vi "Live Capture Functional Stack.8.64bit.vi"() -> ()   [LabVIEW 2014]
uses:
  subvis/Stack Track.ctl
  subvis/Stack_State.ctl
  CameraControlTypeDef.ctl
  Desktop/camtiff/ctiff.llb/__CTIFFNewFileAndStyleUINT16.vi
  Desktop/camtiff/ctiff.llb/__CTIFFAddNewPageUINT16.vi
panel:
  in  "Preview":bool
  in  "Capture Mode":bool
  out "Record Ready":bool
  in  "Stacks":dbl=1.0
  out "Stack Frames":i32=100
  in  "Stack Frames":i32=100
  in  "Temp":path=path "C:/temp.tmp"
  in  "Frames":i32=100
  in  "HardDisk Record":bool
  in  "Internal Line Interval":dbl
  in  "Slit Width / Lines":sgl=150.0
  in  "Camera Readout Mode":u16(ring)=12 items=["Full Frame"=1, "Slit Scanning"=12]
  in  "Readout Direction":sgl(ring)=1.0 items=["Forward"=1, "Backward"=2]
  in  "Trigger Mode":sgl(ring)=1.0 items=["Normal"=1, "Start "=6]
  in  "Trigger Source":sgl(ring)=2.0 items=["Internal"=1, "External"=2]
  out "State":T1=enum."Start Sequence"
  out "Image":u16[][](graph)
  out "Saving":bool
  in  "AutoIncrement":bool=TRUE
  in  "Path":path=path "C:/Users/spim/Desktop/Craig Cap/temp/a.tiff"
  in  "Frames":i32=100
  out "Frame Index":i32
  out "error out":errorcluster
  in  "stop":bool
  in  "Ram Record":bool
  out "Total Frames":i32
  out "Elapsed Time":u32
  out "Software FPS":dbl
  out "Camera FPS":dbl
  in  "H Offset":i32 min=0 max=0 step=4
  in  "H Width":i32 min=0 max=2048 step=4
  out "SMD":dbl
  out "SHO":i32
  in  "V Offset":i32 min=0 max=0 step=4
  in  "V Width":i32 min=0 max=2048 step=4
  in  "Binning":u16(ring) items=["1x1"=1, "2x2"=2, "4x4"=4]
  out "SHW":i32
  out "SVO":i32
  out "SVW":i32
  in  "Scan Mode":dbl min=0.0 max=2.0 step=1.0
  in  "Exposure":dbl min=0.0 max=10.000004210526315 step=1e-08
  out "EXP":dbl
  out "Camera Model":string
  out "Camera Version":string
  out "Camera Serial":string
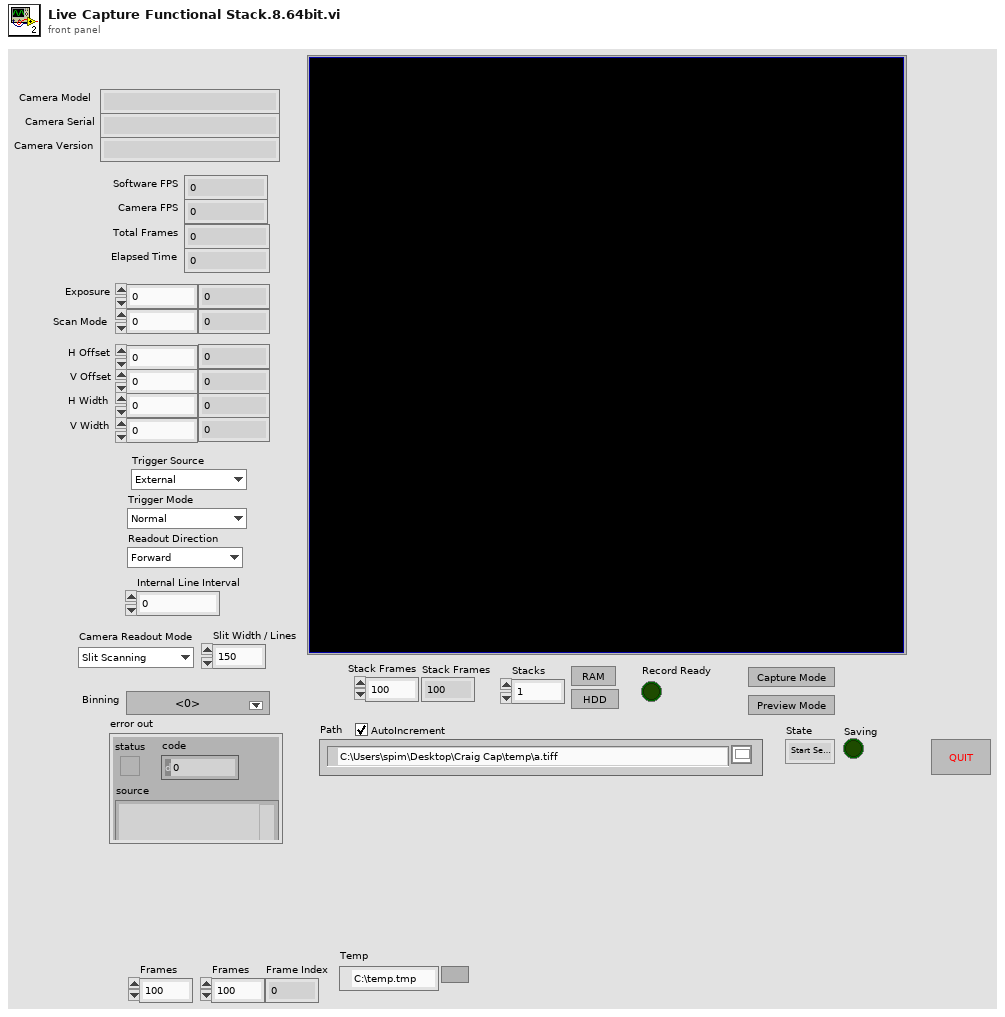
[diagram p1: front panel]
types:
  T1 = typedef "Stack Track.ctl" = enum16{"Idle", "Start Sequence", "Read Disk", "STOP", "Collecting", "End"}
  T2 = typedef "CameraControlTypeDef.ctl" = enum16{"IntervalLineInt", "Ram Record", "HardDisk Record", "Disengage Update", "Update", "Idle", "ROI", "Binning", "Scan Mode", "Trigger Mode", "Readout Mode", "Readout Direction", "Preview"}
  T3 = typedef "Stack_State.ctl" = cluster{"State":T1, "Stack Number":i32, "Image":u16[][]}
  T4 = enum8{"Enabled", "Disabled", "Disabled and Grayed Out"}
  T5 = cluster{"Model":string, "Camera ID":string, "Firmware":string}
  T6 = cluster{"Value":i32, "Minimum":i32, "Maximum":i32, "Increment":i32}
  T7 = cluster{"height":u32, "width":u32, "datatype":u32}
  T8 = cluster{"H Offset":i32, "V Offset":i32, "H Width":i32, "V Width":i32}
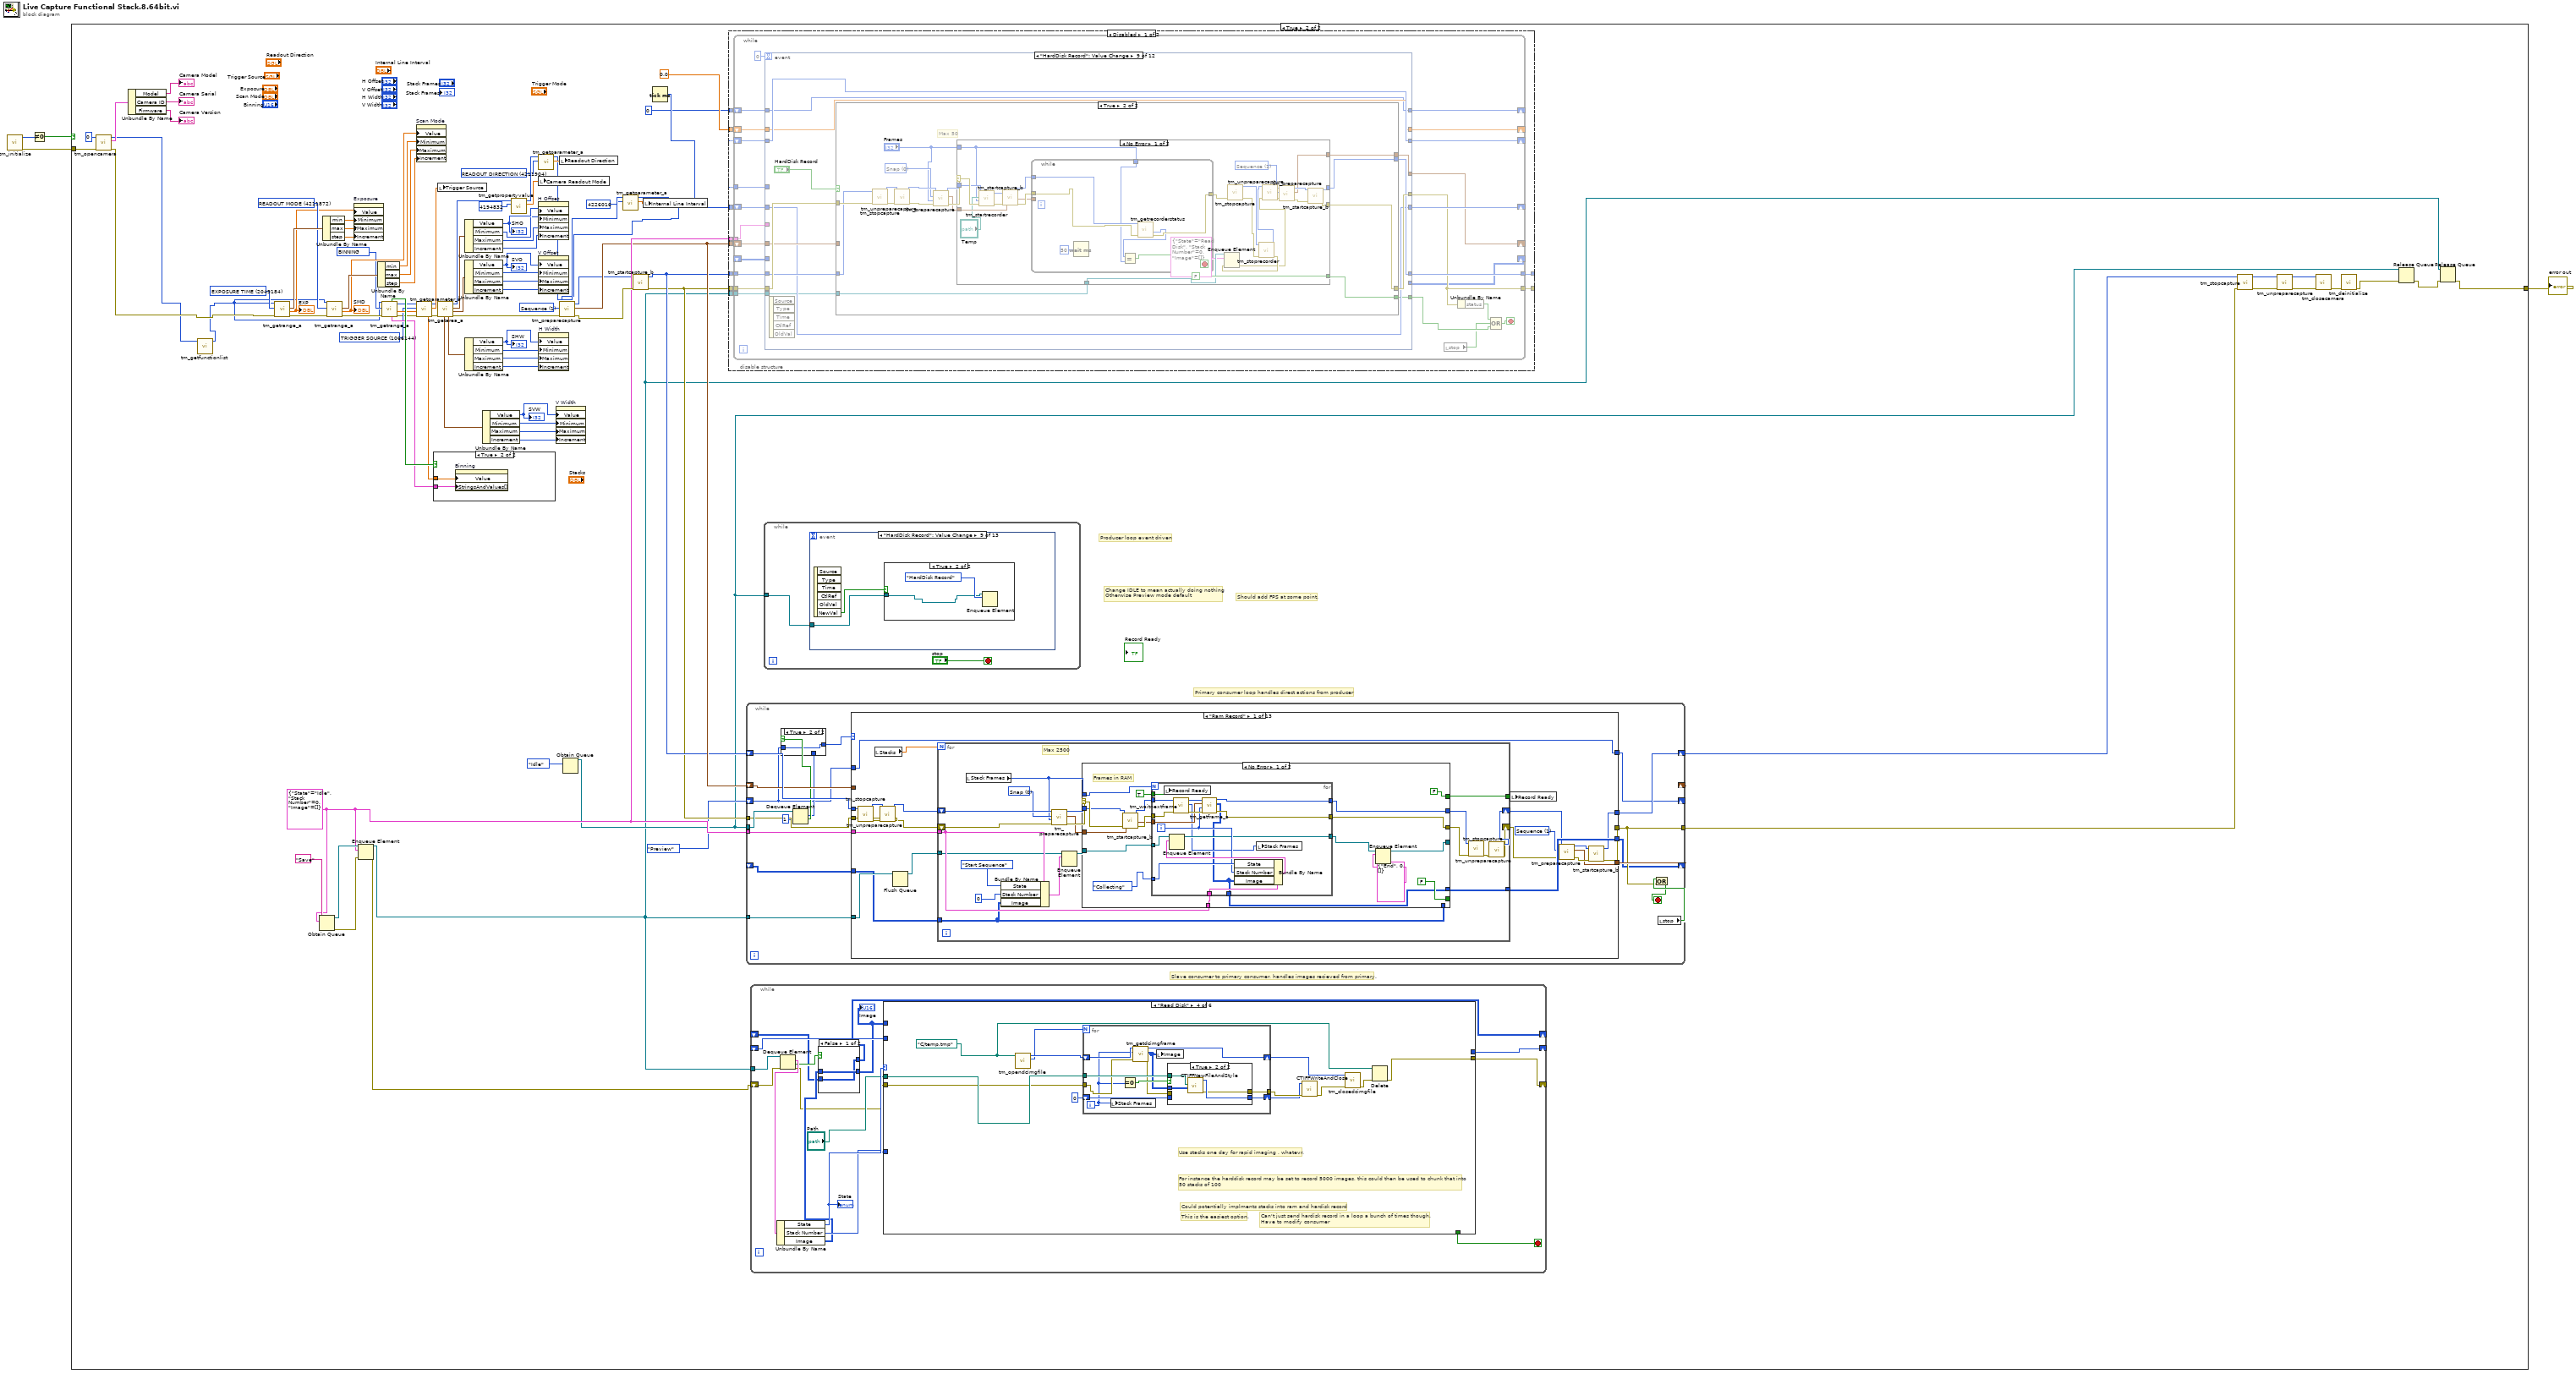
[diagram p0: block diagram]
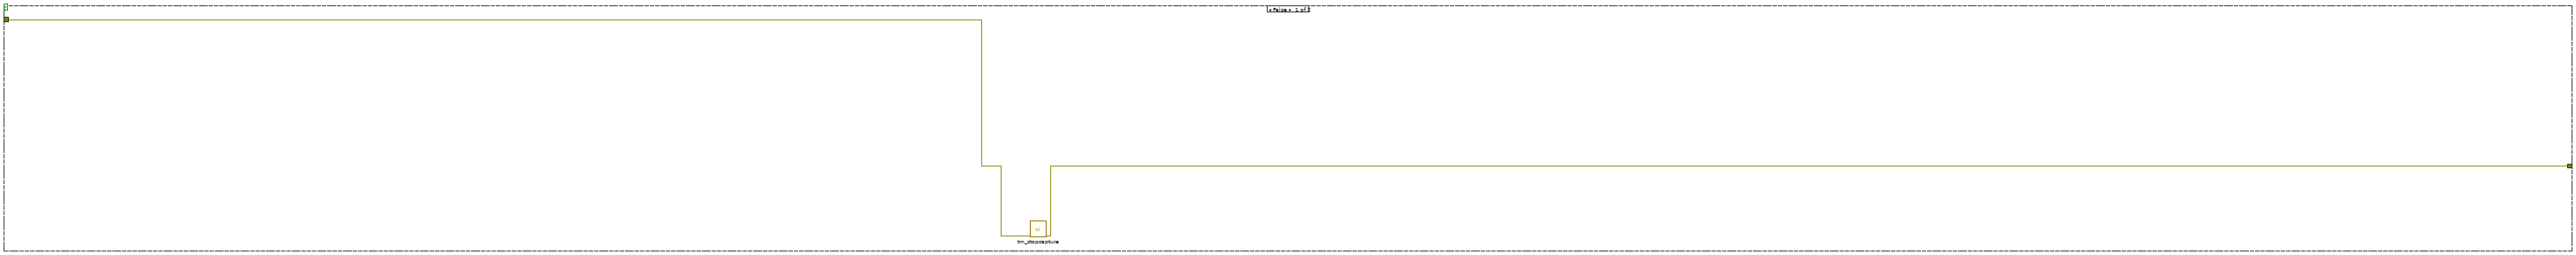
[diagram p2: hidden frame]
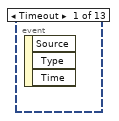
[diagram p3: hidden frame]
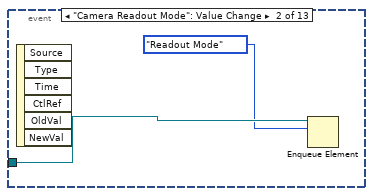
[diagram p4: hidden frame]
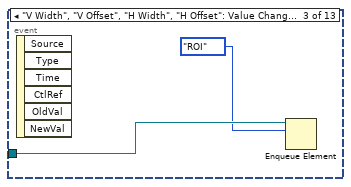
[diagram p5: hidden frame]
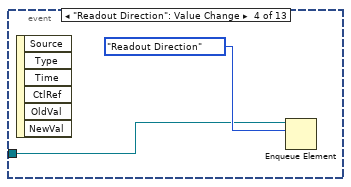
[diagram p6: hidden frame]
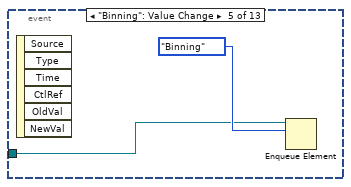
[diagram p7: hidden frame]
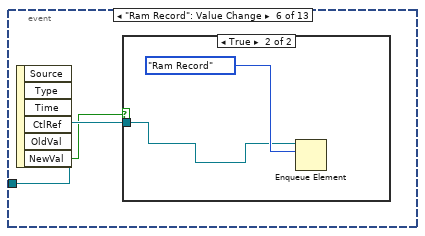
[diagram p8: hidden frame]
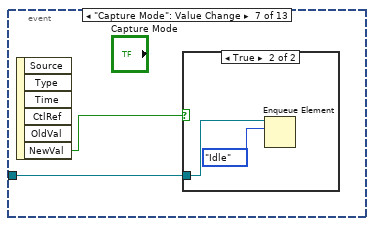
[diagram p10: hidden frame]
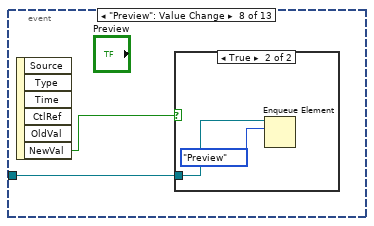
[diagram p12: hidden frame]
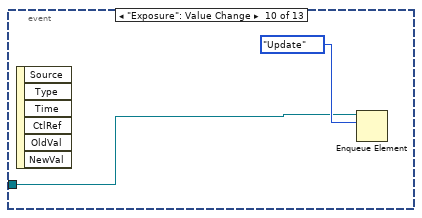
[diagram p15: hidden frame]
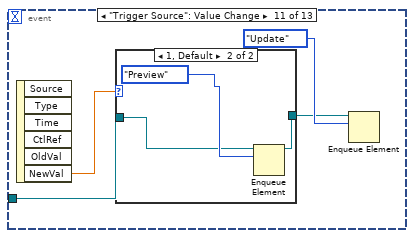
[diagram p16: hidden frame]
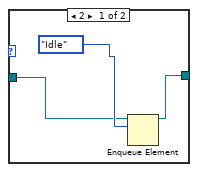
[diagram p17: hidden frame]
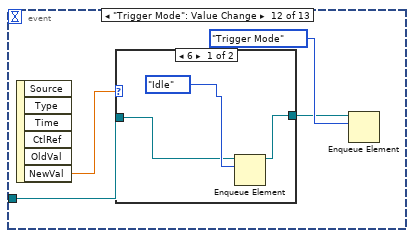
[diagram p18: hidden frame]
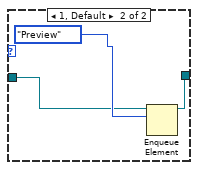
[diagram p19: hidden frame]
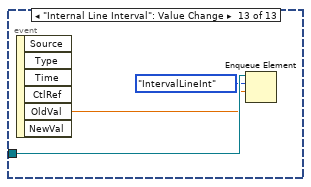
[diagram p20: hidden frame]
diagram:
  n1 = call <userlib>:"tm_initialize.vi"() -> ("error out"=w2:errorcluster, "Number Of Cameras"=w1:u32)  [unwired: 8 in, 2 out]
  n2 = Not Equal To 0?(x=w1) -> (x != 0?=w4:bool)
  n3 = case shown="True" w4 {
    tunnel: [w5 w15] -> w3
    tunnel: w2 -> [w6 w98]
    frame False {
      n4 = call <userlib>:"tm_stopcapture.vi"("error in (no error)"=w6) -> ("error out"=w5:errorcluster)  [unwired: 9 in, 1 out]
    }
    frame True {
      w33 = u32 4211904 items=["SENSOR MODE"=4212128, "CCD MODE"=4212384, "READOUT MODE"=4211872, "ACTIVE VIEW INDEX"=4343136, "BITS PER CHANNEL"=4342976, "IMAGE PIXEL TYPE"=4343296, "BINNING"=4215968, "EXPOSURE TIME"=2049184, "CONTRAST GAIN"=3163312, "CONTRAST OFFSET"=3163328, "LIGHT MODE"=2114720, "SENSITIVITY"=2114992, "PHOTON IMAGING MODE"=2115200, "HIGH DYNAMIC RANGE MODE"=3163360, "WHITE BALANCE"=3163568, "TEMPERATURE"=2115232, "TEMPERATURE TARGET"=2115264, "SENSOR COOLER FAN"=2115296, "LINEBUNDLE HEIGHT"=4212192, "MECHANICAL SHUTTER"=2115488, "BACK FOCUS POSITION"=8422304, "TRIGGER CONNECTOR"=1066432, "TRIGGER SOURCE"=1066144, "OUTPUT TRIGGER SOURCE"=1852576, "TRIGGER GLOBAL EXPOSURE"=2049680, "FIRST TRIGGER BEHAVIOR"=2049696, "CHANNEL SYNC"=1852352, "READOUT DIRECTION"=4211904, "PRE HSYNC COUNT"=1852704] ("Parameter")
      w42 = u32 1066144 items=["SENSOR MODE"=4212128, "CCD MODE"=4212384, "READOUT MODE"=4211872, "ACTIVE VIEW INDEX"=4343136, "BITS PER CHANNEL"=4342976, "IMAGE PIXEL TYPE"=4343296, "BINNING"=4215968, "EXPOSURE TIME"=2049184, "CONTRAST GAIN"=3163312, "CONTRAST OFFSET"=3163328, "LIGHT MODE"=2114720, "SENSITIVITY"=2114992, "PHOTON IMAGING MODE"=2115200, "HIGH DYNAMIC RANGE MODE"=3163360, "WHITE BALANCE"=3163568, "TEMPERATURE"=2115232, "TEMPERATURE TARGET"=2115264, "SENSOR COOLER FAN"=2115296, "LINEBUNDLE HEIGHT"=4212192, "MECHANICAL SHUTTER"=2115488, "BACK FOCUS POSITION"=8422304, "TRIGGER CONNECTOR"=1066432, "TRIGGER SOURCE"=1066144, "OUTPUT TRIGGER SOURCE"=1852576, "TRIGGER GLOBAL EXPOSURE"=2049680, "FIRST TRIGGER BEHAVIOR"=2049696, "CHANNEL SYNC"=1852352, "READOUT DIRECTION"=4211904, "PRE HSYNC COUNT"=1852704] ("Parameter")
      w28 = T3 {"State"=enum."Idle", "Stack Number"=0, "Image"=[]} ("input cluster")
      w47 = u32 2049184 items=["BINNING"=4215968, "BITS PER CHANNEL"=4342976, "ACTIVE VIEW INDEX"=4343136, "CCD MODE"=4212384, "SENSOR MODE"=4212128, "READOUT MODE"=4211872, "EXPOSURE TIME"=2049184, "CONTRAST GAIN"=3163312, "CONTRAST OFFSET"=3163328, "LIGHT MODE"=2114720, "SENSITIVITY"=2114992, "WHITE BALANCE"=3163568, "PHOTON IMAGING MODE"=2115200, "HIGH DYNAMIC RANGE MODE"=3163360, "TRIGGER SOURCE"=1066144, "TRIGGER ACTIVE"=1066160, "TRIGGER MODE"=1066400, "TRIGGER POLARITY"=1066416, "TRIGGER GLOBAL EXPOSURE"=2049680, "FIRST TRIGGER BEHAVIOR"=2049696, "TRIGGER TIMES"=1066448, "OUTPUT TRIGGER POLARITY"=1852592, "OUTPUT TRIGGER DELAY"=1852624, "OUTPUT TRIGGER PERIOD"=1852640, "TEMPERATURE"=2115232, "TEMPERATURE TARGET"=2115264, "SENSOR COOLER FAN"=2115296, "MECHANICAL SHUTTER"=2115488, "BACK FOCUS POSITION"=8422304, "FRAMEBUNDLE MODE"=4346784, "FRAMEBUNDLE NUMBER"=4346800, "LINEBUNDLE HEIGHT"=4212192, "TRIGGER CONNECTOR"=1066432, "IMAGE PIXEL TYPE"=4343296, "OUTPUT TRIGGER KIND"=1852656, "READOUT DIRECTION"=4211904, "CHANNEL SYNC"=1852352] ("Parameter")
      w48 = u32 4211872 items=["BINNING"=4215968, "BITS PER CHANNEL"=4342976, "ACTIVE VIEW INDEX"=4343136, "CCD MODE"=4212384, "SENSOR MODE"=4212128, "READOUT MODE"=4211872, "EXPOSURE TIME"=2049184, "CONTRAST GAIN"=3163312, "CONTRAST OFFSET"=3163328, "LIGHT MODE"=2114720, "SENSITIVITY"=2114992, "WHITE BALANCE"=3163568, "PHOTON IMAGING MODE"=2115200, "HIGH DYNAMIC RANGE MODE"=3163360, "TRIGGER SOURCE"=1066144, "TRIGGER ACTIVE"=1066160, "TRIGGER MODE"=1066400, "TRIGGER POLARITY"=1066416, "TRIGGER GLOBAL EXPOSURE"=2049680, "FIRST TRIGGER BEHAVIOR"=2049696, "TRIGGER TIMES"=1066448, "OUTPUT TRIGGER POLARITY"=1852592, "OUTPUT TRIGGER DELAY"=1852624, "OUTPUT TRIGGER PERIOD"=1852640, "TEMPERATURE"=2115232, "TEMPERATURE TARGET"=2115264, "SENSOR COOLER FAN"=2115296, "MECHANICAL SHUTTER"=2115488, "BACK FOCUS POSITION"=8422304, "FRAMEBUNDLE MODE"=4346784, "FRAMEBUNDLE NUMBER"=4346800, "LINEBUNDLE HEIGHT"=4212192, "TRIGGER CONNECTOR"=1066432, "IMAGE PIXEL TYPE"=4343296, "OUTPUT TRIGGER KIND"=1852656, "READOUT DIRECTION"=4211904, "CHANNEL SYNC"=1852352] ("Parameter")
      w49 = u32 4215968 items=["BINNING"=4215968, "BITS PER CHANNEL"=4342976, "ACTIVE VIEW INDEX"=4343136, "CCD MODE"=4212384, "SENSOR MODE"=4212128, "READOUT MODE"=4211872, "EXPOSURE TIME"=2049184, "CONTRAST GAIN"=3163312, "CONTRAST OFFSET"=3163328, "LIGHT MODE"=2114720, "SENSITIVITY"=2114992, "WHITE BALANCE"=3163568, "PHOTON IMAGING MODE"=2115200, "HIGH DYNAMIC RANGE MODE"=3163360, "TRIGGER SOURCE"=1066144, "TRIGGER ACTIVE"=1066160, "TRIGGER MODE"=1066400, "TRIGGER POLARITY"=1066416, "TRIGGER GLOBAL EXPOSURE"=2049680, "FIRST TRIGGER BEHAVIOR"=2049696, "TRIGGER TIMES"=1066448, "OUTPUT TRIGGER POLARITY"=1852592, "OUTPUT TRIGGER DELAY"=1852624, "OUTPUT TRIGGER PERIOD"=1852640, "TEMPERATURE"=2115232, "TEMPERATURE TARGET"=2115264, "SENSOR COOLER FAN"=2115296, "MECHANICAL SHUTTER"=2115488, "BACK FOCUS POSITION"=8422304, "FRAMEBUNDLE MODE"=4346784, "FRAMEBUNDLE NUMBER"=4346800, "LINEBUNDLE HEIGHT"=4212192, "TRIGGER CONNECTOR"=1066432, "IMAGE PIXEL TYPE"=4343296, "OUTPUT TRIGGER KIND"=1852656, "READOUT DIRECTION"=4211904, "CHANNEL SYNC"=1852352] ("Parameter")
      w94 = 1 items=["Snap", "Sequence"] ("Capture mode")
      # "Change IDLE to mean actually doing nothing\nOtherwise Preview mode default"
      # "Slave consumer to primary consumer, handles images recieved from primary."
      # "Primary consumer loop handles direct actions from producer"
      # "Producer loop event driven"
      # "Should add FPS at some point."
      n5 = call <userlib>:"tm_opencamera.vi"("error in (no error)"=w98, "Camera Index"=u32 0) -> ("error out"=w29:errorcluster, "Camera Details"=w61:T5, "Handle out"=w13:u32)  [unwired: 7 in]
      n6 = Unbundle By Name(w61) -> ("Model"=→"Camera Model":string, "Camera ID"=→"Camera Serial":string, "Firmware"=→"Camera Version":string)
      n7 = call <userlib>:"tm_getfunctionlist.vi"("Handle in"=w13) -> ("Handle out"=w12:u32)  [unwired: 8 in, 2 out]
      n8 = call <userlib>:"tm_getrange_a.vi"("error in (no error)"=w29, "Parameter"=w47, "Handle in"=w12) -> ("error out"=w56:errorcluster, "default"=w45:dbl, "Range"=w57:cluster{"min":dbl, "max":dbl, "step":dbl})  [unwired: 2 in, 4 out]
      "EXP" <- w45
      n9 = Obtain Queue(name (unnamed)="Save", element data type=w28) -> (queue out=w31:refnum<queue>, error out=w10:errorcluster)  [unwired: 3 in, 1 out]
      n10 = Unbundle By Name(w57) -> ("min"=w92:dbl, "max"=w91:dbl, "step"=w90:dbl)
      n11 = call <userlib>:"tm_getrange_a.vi"("error in (no error)"=w56, "Parameter"=w48, "Handle in"=w12) -> ("error out"=w53:errorcluster, "default"=w54:dbl, "Range"=w55:cluster{"min":dbl, "max":dbl, "step":dbl})  [unwired: 2 in, 4 out]
      "SMD" <- w54
      n12 = property on="Exposure" class="DigNum (strict)"("Value"=w45, "Minimum"=w92, "Maximum"=w91, "Increment"=w90) -> ()  [unwired: 2 in, 2 out]
      n13 = Enqueue Element(queue=w31, element=w28, error in (no error)=w10) -> (queue out=w14:refnum<queue>, error out=w9:errorcluster)  [unwired: 1 in, 1 out]
      n14 = Unbundle By Name(w55) -> ("min"=w89:dbl, "max"=w88:dbl, "step"=w87:dbl)
      n15 = call <userlib>:"tm_getrange_a.vi"("error in (no error)"=w53, "Parameter"=w49, "Handle in"=w12) -> ("error out"=w39:errorcluster, "default"=w51:dbl, "Handle out"=w41:u32, "Value Names"=w50:cluster{"Name":string, "Value":dbl}[], "Writable"=w52:bool)  [unwired: 2 in, 2 out]
      n16 = property on="Scan Mode" class="DigNum (strict)"("Value"=w54, "Minimum"=w89, "Maximum"=w88, "Increment"=w87) -> ()  [unwired: 2 in, 2 out]
      n17 = call <userlib>:"tm_getparameter_a.vi"("error in (no error)"=w39, "Parameter"=w42, "Handle in"=w41) -> ("error out"=w38:errorcluster, "Value out"=w43:dbl, "Handle out"=w40:u32)  [unwired: 6 in]
      n18 = case shown="True" w52 {
        tunnel: w50 -> [_ w1167]
        tunnel: w51 -> [_ w1166]
        frame False {
        }
        frame True {
          n19 = property on="Binning" class="Ring (strict)"("Value"=w1166, "StringsAndValues[]"=w1167) -> ()  [unwired: 2 in, 2 out]
        }
      }
      n20 = local write "Trigger Source"(w43) -> ()
      n21 = call <userlib>:"tm_getarea_a.vi"("error in (no error)"=w38, "Handle in"=w40) -> ("error out"=w44:errorcluster, "V Offset"=w86:T6, "H Offset"=w67:T6, "Handle out"=w35:u32, "H Width"=w85:T6, "V Width"=w84:T6)  [unwired: 4 in]
      n22 = Unbundle By Name(w67) -> ("Value"=w66:i32, "Minimum"=w65:i32, "Maximum"=w64:i32, "Increment"=w63:i32)
      "SHO" <- w66
      n23 = Unbundle By Name(w86) -> ("Value"=w74:i32, "Minimum"=w83:i32, "Maximum"=w82:i32, "Increment"=w81:i32)
      "SVO" <- w74
      n24 = Unbundle By Name(w85) -> ("Value"=w73:i32, "Minimum"=w80:i32, "Maximum"=w79:i32, "Increment"=w78:i32)
      "SHW" <- w73
      n25 = Unbundle By Name(w84) -> ("Value"=w72:i32, "Minimum"=w77:i32, "Maximum"=w76:i32, "Increment"=w75:i32)
      "SVW" <- w72
      n26 = call <userlib>:"tm_getpropertyvalue.vi"("Property ID"=u32 4194832, "Handle in"=w35) -> ("Value in"=w36:sgl, "Handle out"=w34:u32)  [unwired: 7 in, 1 out]
      n27 = call <userlib>:"tm_getparameter_a.vi"("Parameter"=w33, "Handle in"=w34) -> ("Value out"=w32:dbl, "Handle out"=w19:u32)  [unwired: 7 in, 1 out]
      n28 = local write "Camera Readout Mode"(w36) -> ()
      n29 = property on="H Offset" class="DigNum (strict)"("Value"=w66, "Minimum"=w65, "Maximum"=w64, "Increment"=w63) -> ()  [unwired: 2 in, 2 out]
      n30 = property on="V Offset" class="DigNum (strict)"("Value"=w74, "Minimum"=w83, "Maximum"=w82, "Increment"=w81) -> ()  [unwired: 2 in, 2 out]
      n31 = property on="H Width" class="DigNum (strict)"("Value"=w73, "Minimum"=w80, "Maximum"=w79, "Increment"=w78) -> ()  [unwired: 2 in, 2 out]
      n32 = property on="V Width" class="DigNum (strict)"("Value"=w72, "Minimum"=w77, "Maximum"=w76, "Increment"=w75) -> ()  [unwired: 2 in, 2 out]
      n33 = local write "Readout Direction"(w32) -> ()
      n34 = Obtain Queue(element data type=CameraControlTypeDef."Idle" ("Enum")) -> (queue out=w17:refnum<queue>)  [unwired: 4 in, 2 out]
      n35 = call <userlib>:"tm_getparameter_a.vi"("Parameter"=4226016, "Handle in"=w19) -> ("Value out"=w7:dbl, "Handle out"=w8:u32)  [unwired: 7 in, 1 out]
      n36 = call <userlib>:"tm_preparecapture.vi"("error in (no error)"=w44, "Capture mode"=w94, "Handle in"=w8) -> ("error out"=w30:errorcluster, "Buffer Info"=w27:T7, "Handle out"=w20:u32)  [unwired: 5 in, 1 out]
      n37 = call <userlib>:"tm_startcapture_b.vi"("error in (no error)"=w30, "Handle in"=w20) -> ("error out"=w25:errorcluster, "Handle out"=w26:u32)  [unwired: 8 in]
      n38 = local write "Internal Line Interval"(w7) -> ()
      n39 = Tick Count (ms)() -> (millisecond timer value=w93:u32)
      n40 = disable-structure shown="Disabled" {
        disable-tunnel: 0.0 -> [w582 _]
        disable-tunnel: w93 -> [w581 _]
        disable-tunnel: 0 -> [w580 _]
        disable-tunnel: [w579 _] -> _
        disable-tunnel: [w578 _] -> _
        disable-tunnel: w28 -> [w577 _]
        disable-tunnel: w27 -> [w576 _]
        disable-tunnel: w26 -> [w575 _]
        disable-tunnel: w25 -> [w574 _]
        disable-tunnel: w14 -> [w573 _]
        frame Disabled {
          n41 = while {
            tunnel: w574 -> [w596]
            tunnel: [w594] -> w578
            tunnel: [w593] -> w579
            shift-right: [w603] -> _
            shift-left: w581 -> [w601]
            shift-right: [w604] -> _
            shift-left: w582 -> [w602]
            shift-right: [w595] -> _
            shift-left: w581 -> [w599]
            tunnel: w575 -> [w597]
            tunnel: w581 -> [w600]
            shift-right: [w592] -> _
            shift-left: w576 -> [w598]
            shift-right: [w590] -> _
            shift-left: w580 -> [w591]
            tunnel: w573 -> [w589]
            shift-right: [w587] -> _
            shift-left: _ -> [w586]
            tunnel: w577 -> [w585]
            stop <- w605 stop-if-true
            n42 = event shown="[8] \"HardDisk Record\": Value Change" {
              selector: _ -> [_ _ _ _ _ _ _ _ _ _ _ _]
              dyn-events: _ -> [_ _ _ _ _ _ _ _ _ _ _ _]
              timeout: 0 -> [_ _ _ _ _ _ _ _ _ _ _ _]
              tunnel: [w616 w685 w699 w712 w731 w751 w773 w801 w898 w992 w1028 w1073] -> w604
              tunnel: [w615 w686 w700 w713 w732 w752 w774 w802 w899 w993 w1029 w1074] -> w603
              tunnel: w602 -> [w627 w685 w699 w712 w731 w751 w773 w801 w898 w992 w1028 w1073]
              tunnel: w601 -> [w618 w686 w700 w713 w732 w752 w774 w802 w899 w993 w1029 w1074]
              tunnel: w600 -> [w623 _ _ _ _ _ _ _ _ _ _ _]
              tunnel: w599 -> [w628 w687 w701 w714 w733 w753 w775 w797 w894 w994 w1036 w1081]
              tunnel: w598 -> [w622 w684 w698 w711 _ w750 _ w798 w895 _ _ _]
              tunnel: w597 -> [w630 w680 w693 w707 w726 w744 w766 w805 w902 w989 w1005 w1043]
              tunnel: w596 -> [w629 w682 w689 w708 w725 w747 w765 w806 w903 w988 w1004 w1042]
              tunnel: [w626 w687 w701 w714 w733 w753 w775 w797 w894 w994 w1036 w1081] -> w595
              tunnel: [w625 w677 w696 w704 w717 w737 w756 w803 w900 w983 w1031 w1076] -> w594
              tunnel: [w624 w676 w695 w703 w716 w736 w754 w804 w901 w984 w1032 w1077] -> w593
              tunnel: [w621 w684 w698 w711 w720 w750 w761 w799 w896 w982 w1030 w1075] -> w592
              tunnel: w591 -> [w613 w683 w697 w710 w730 w749 w772 w800 w897 w981 w1001 w1037]
              tunnel: [w612 w683 w697 w710 w730 w749 w772 w800 w897 w981 w1001 w1037] -> w590
              tunnel: w589 -> [w607 _ _ _ _ _ _ w796 w893 _ _ _]
              tunnel: [_ _ _ _ _ _ _ w795 w892 _ _ _] -> w588
              tunnel: w585 -> [w610 _ _ _ _ _ _ w793 _ _ _ _]
              tunnel: [w609 _ _ _ _ _ _ _ _ _ _ _] -> w587
              tunnel: w586 -> [w608 _ _ _ _ _ _ w794 _ _ _ _]
              event Timeout {
                n43 = event-data() -> ()  [unwired: 1 in, 2 out]
                n44 = call <userlib>:"tm_waitnextframe.vi"("error in (no error)"=w629, "Handle in"=w630) -> ("error out"=w633:errorcluster, "Frame Count"=w614:i32, "Frame Index"=w632:i32, "Handle out"=w634:u32)  [unwired: 6 in]
                "Total Frames" <- w614
                n45 = Tick Count (ms)() -> (millisecond timer value=w620:u32)
                n46 = Increment(x=w627) -> (x+1=w617:dbl)
                n47 = Subtract(x=w620, y=w623) -> (x-y=→"Elapsed Time":u32)
                n48 = Add(x=w618, y=u32 1000) -> (x+y=w638:u32)
                n49 = Less Or Equal?(x=w638, y=w620) -> (x <= y?=w619:bool)
                n50 = Add(x=w628, y=u32 50) -> (x+y=w636:u32)
                n51 = Less Or Equal?(x=w636, y=w620) -> (x <= y?=w611:bool)
                n52 = case shown="True" w619 {
                  tunnel: w618 -> [w641 w650]
                  tunnel: [w641 w647] -> w615
                  tunnel: w617 -> [w640 w653]
                  tunnel: w620 -> [_ w647]
                  tunnel: [w640 0.0] -> w616
                  tunnel: w614 -> [_ w642]
                  tunnel: w613 -> [w639 w645]
                  tunnel: [w639 w642] -> w612
                  frame False {
                  }
                  frame True {
                    n53 = Subtract(x=w647, y=w650) -> (x-y=w649:u32)
                    n54 = Subtract(x=w642, y=w645) -> (x-y=w643:i32)
                    n55 = To Double Precision Float(number=w649) -> (double precision float=w655:dbl)
                    n56 = Divide(x=w655, y=1000.0) -> (x/y=w646:dbl)
                    n57 = To Double Precision Float(number=w643) -> (double precision float=w644:dbl)
                    n58 = Divide(x=w644, y=w646) -> (x/y=→"Camera FPS":dbl)
                    n59 = Divide(x=w653, y=w646) -> (x/y=→"Software FPS":dbl)
                  }
                }
                n60 = case shown="True" w611 {
                  tunnel: w628 -> [w660 _]
                  tunnel: w620 -> [_ w673]
                  tunnel: [w660 w673] -> w626
                  tunnel: w634 -> [w659 w672]
                  tunnel: w622 -> [w657 w667]
                  tunnel: w633 -> [w658 w671]
                  tunnel: [w659 w670] -> w625
                  tunnel: [w658 w669] -> w624
                  tunnel: w632 -> [_ w668]
                  tunnel: [w657 w667] -> w621
                  tunnel: w607 -> [_ w666]
                  tunnel: w610 -> [_ w662]
                  tunnel: [w656 w661] -> w609
                  tunnel: w608 -> [w656 _]
                  frame False {
                  }
                  frame True {
                    n61 = call <userlib>:"tm_getframe_a.vi"("error in (no error)"=w671, "Frame Index"=w668, "Buffer Info"=w667, "Handle in"=w672) -> ("error out"=w669:errorcluster, "Data 16"=w661:u16[][], "Handle out"=w670:u32)  [unwired: 3 in, 2 out]
                    n62 = Bundle By Name(cluster=w662, "State"=Stack_Track."Idle", "Stack Number"=0, "Image"=w661) -> (w663:T3)
                    n63 = Enqueue Element(queue=w666, element=w663) -> ()  [unwired: 2 in, 3 out]
                  }
                }
              }
              event "Exposure": Value Change {
                w675 = u32 2049184 items=["SENSOR MODE"=4212128, "CCD MODE"=4212384, "READOUT MODE"=4211872, "ACTIVE VIEW INDEX"=4343136, "BITS PER CHANNEL"=4342976, "IMAGE PIXEL TYPE"=4343296, "BINNING"=4215968, "EXPOSURE TIME"=2049184, "CONTRAST GAIN"=3163312, "CONTRAST OFFSET"=3163328, "LIGHT MODE"=2114720, "SENSITIVITY"=2114992, "PHOTON IMAGING MODE"=2115200, "HIGH DYNAMIC RANGE MODE"=3163360, "WHITE BALANCE"=3163568, "TEMPERATURE"=2115232, "TEMPERATURE TARGET"=2115264, "SENSOR COOLER FAN"=2115296, "LINEBUNDLE HEIGHT"=4212192, "MECHANICAL SHUTTER"=2115488, "BACK FOCUS POSITION"=8422304, "TRIGGER CONNECTOR"=1066432, "TRIGGER SOURCE"=1066144, "OUTPUT TRIGGER SOURCE"=1852576, "TRIGGER GLOBAL EXPOSURE"=2049680, "FIRST TRIGGER BEHAVIOR"=2049696, "CHANNEL SYNC"=1852352, "READOUT DIRECTION"=4211904, "PRE HSYNC COUNT"=1852704] ("Parameter")
                n64 = event-data() -> ("NewVal"=w681:dbl)  [unwired: 1 in, 2 out]
                n65 = call <userlib>:"tm_setparameter_a.vi"("error in (no error)"=w682, "Value in"=w681, "Parameter"=w675, "Handle in"=w680) -> ("error out"=w679:errorcluster, "Handle out"=w678:u32)  [unwired: 6 in]
                n66 = call <userlib>:"tm_getparameter_a.vi"("error in (no error)"=w679, "Parameter"=w675, "Handle in"=w678) -> ("error out"=w676:errorcluster, "Value out"=w674:dbl, "Handle out"=w677:u32)  [unwired: 6 in]
                n67 = local write "EXP"(w674) -> ()
              }
              event "Internal Line Interval": Value Change {
                w688 = u32 4191424 items=["SENSOR MODE"=4212128, "CCD MODE"=4212384, "READOUT MODE"=4211872, "ACTIVE VIEW INDEX"=4343136, "BITS PER CHANNEL"=4342976, "IMAGE PIXEL TYPE"=4343296, "BINNING"=4215968, "EXPOSURE TIME"=2049184, "CONTRAST GAIN"=3163312, "CONTRAST OFFSET"=3163328, "LIGHT MODE"=2114720, "SENSITIVITY"=2114992, "PHOTON IMAGING MODE"=2115200, "HIGH DYNAMIC RANGE MODE"=3163360, "WHITE BALANCE"=3163568, "TEMPERATURE"=2115232, "TEMPERATURE TARGET"=2115264, "SENSOR COOLER FAN"=2115296, "LINEBUNDLE HEIGHT"=4212192, "MECHANICAL SHUTTER"=2115488, "BACK FOCUS POSITION"=8422304, "TRIGGER CONNECTOR"=1066432, "TRIGGER SOURCE"=1066144, "OUTPUT TRIGGER SOURCE"=1852576, "TRIGGER GLOBAL EXPOSURE"=2049680, "FIRST TRIGGER BEHAVIOR"=2049696, "CHANNEL SYNC"=1852352, "READOUT DIRECTION"=4211904, "PRE HSYNC COUNT"=1852704, "INTERNAL LINE SPEED"=4191408, "INTERNAL LINE INVERVAL"=4191424] ("Parameter")
                n68 = event-data() -> ("NewVal"=w692:dbl)  [unwired: 1 in, 2 out]
                n69 = call <userlib>:"tm_setparameter_a.vi"("error in (no error)"=w689, "Value in"=w692, "Parameter"=w688, "Handle in"=w693) -> ("error out"=w690:errorcluster, "Handle out"=w691:u32)  [unwired: 6 in]
                n70 = call <userlib>:"tm_getparameter_a.vi"("error in (no error)"=w690, "Parameter"=w688, "Handle in"=w691) -> ("error out"=w695:errorcluster, "Value out"=w694:dbl, "Handle out"=w696:u32)  [unwired: 6 in]
                n71 = local write "Internal Line Interval"(w694) -> ()
              }
              event "Trigger Source": Value Change {
                w709 = u32 1066144 items=["SENSOR MODE"=4212128, "CCD MODE"=4212384, "READOUT MODE"=4211872, "ACTIVE VIEW INDEX"=4343136, "BITS PER CHANNEL"=4342976, "IMAGE PIXEL TYPE"=4343296, "BINNING"=4215968, "EXPOSURE TIME"=2049184, "CONTRAST GAIN"=3163312, "CONTRAST OFFSET"=3163328, "LIGHT MODE"=2114720, "SENSITIVITY"=2114992, "PHOTON IMAGING MODE"=2115200, "HIGH DYNAMIC RANGE MODE"=3163360, "WHITE BALANCE"=3163568, "TEMPERATURE"=2115232, "TEMPERATURE TARGET"=2115264, "SENSOR COOLER FAN"=2115296, "LINEBUNDLE HEIGHT"=4212192, "MECHANICAL SHUTTER"=2115488, "BACK FOCUS POSITION"=8422304, "TRIGGER CONNECTOR"=1066432, "TRIGGER SOURCE"=1066144, "OUTPUT TRIGGER SOURCE"=1852576, "TRIGGER GLOBAL EXPOSURE"=2049680, "FIRST TRIGGER BEHAVIOR"=2049696, "CHANNEL SYNC"=1852352, "READOUT DIRECTION"=4211904, "PRE HSYNC COUNT"=1852704] ("Parameter")
                n72 = event-data() -> ("NewVal"=w702:sgl)  [unwired: 1 in, 3 out]
                n73 = call <userlib>:"tm_setparameter_a.vi"("error in (no error)"=w708, "Value in"=w702, "Parameter"=w709, "Handle in"=w707) -> ("error out"=w706:errorcluster, "Handle out"=w705:u32)  [unwired: 6 in]
                n74 = call <userlib>:"tm_getparameter_a.vi"("error in (no error)"=w706, "Parameter"=w709, "Handle in"=w705) -> ("error out"=w703:errorcluster, "Handle out"=w704:u32)  [unwired: 6 in, 1 out]
              }
              event "Trigger Mode": Value Change {
                w721 = 1 items=["Snap", "Sequence"] ("Capture mode")
                n75 = event-data() -> ("NewVal"=w715:sgl)  [unwired: 1 in, 4 out]
                n76 = call <userlib>:"tm_stopcapture.vi"("error in (no error)"=w725, "Handle in"=w726) -> ("error out"=w728:errorcluster, "Handle out"=w727:u32)  [unwired: 8 in]
                n77 = call <userlib>:"tm_unpreparecapture.vi"("error in (no error)"=w728, "Handle in"=w727) -> ("error out"=w724:errorcluster, "Handle out"=w723:u32)  [unwired: 8 in]
                n78 = call <userlib>:"tm_setpropertyvalue.vi"("error in (no error)"=w724, "Value in"=w715, "Property ID"=u32 1049104, "Handle in"=w723) -> ("error out"=w719:errorcluster, "Handle out"=w722:u32)  [unwired: 6 in]
                n79 = call <userlib>:"tm_preparecapture.vi"("Capture mode"=w721, "Handle in"=w722) -> ("Buffer Info"=w720:T7, "Handle out"=w718:u32)  [unwired: 6 in, 2 out]
                n80 = call <userlib>:"tm_startcapture_b.vi"("error in (no error)"=w719, "Handle in"=w718) -> ("error out"=w716:errorcluster, "Handle out"=w717:u32)  [unwired: 8 in]
              }
              event "Readout Direction": Value Change {
                w742 = 1 items=["Snap", "Sequence"] ("Capture mode")
                w735 = u32 4211904 items=["SENSOR MODE"=4212128, "CCD MODE"=4212384, "READOUT MODE"=4211872, "ACTIVE VIEW INDEX"=4343136, "BITS PER CHANNEL"=4342976, "IMAGE PIXEL TYPE"=4343296, "BINNING"=4215968, "EXPOSURE TIME"=2049184, "CONTRAST GAIN"=3163312, "CONTRAST OFFSET"=3163328, "LIGHT MODE"=2114720, "SENSITIVITY"=2114992, "PHOTON IMAGING MODE"=2115200, "HIGH DYNAMIC RANGE MODE"=3163360, "WHITE BALANCE"=3163568, "TEMPERATURE"=2115232, "TEMPERATURE TARGET"=2115264, "SENSOR COOLER FAN"=2115296, "LINEBUNDLE HEIGHT"=4212192, "MECHANICAL SHUTTER"=2115488, "BACK FOCUS POSITION"=8422304, "TRIGGER CONNECTOR"=1066432, "TRIGGER SOURCE"=1066144, "OUTPUT TRIGGER SOURCE"=1852576, "TRIGGER GLOBAL EXPOSURE"=2049680, "FIRST TRIGGER BEHAVIOR"=2049696, "CHANNEL SYNC"=1852352, "READOUT DIRECTION"=4211904, "PRE HSYNC COUNT"=1852704] ("Parameter")
                n81 = event-data() -> ("NewVal"=w734:sgl)  [unwired: 1 in, 3 out]
                n82 = call <userlib>:"tm_stopcapture.vi"("error in (no error)"=w747, "Handle in"=w744) -> ("error out"=w748:errorcluster, "Handle out"=w743:u32)  [unwired: 8 in]
                n83 = call <userlib>:"tm_unpreparecapture.vi"("error in (no error)"=w748, "Handle in"=w743) -> ("error out"=w746:errorcluster, "Handle out"=w745:u32)  [unwired: 8 in]
                n84 = call <userlib>:"tm_setparameter_a.vi"("error in (no error)"=w746, "Value in"=w734, "Parameter"=w735, "Handle in"=w745) -> ("error out"=w739:errorcluster, "Handle out"=w738:u32)  [unwired: 6 in]
                n85 = call <userlib>:"tm_preparecapture.vi"("error in (no error)"=w739, "Capture mode"=w742, "Handle in"=w738) -> ("error out"=w740:errorcluster, "Handle out"=w741:u32)  [unwired: 5 in, 2 out]
                n86 = call <userlib>:"tm_startcapture_b.vi"("error in (no error)"=w740, "Handle in"=w741) -> ("error out"=w736:errorcluster, "Handle out"=w737:u32)  [unwired: 8 in]
              }
              event "Camera Readout Mode", "Slit Width / Lines": Value Change {
                w759 = 1 items=["Snap", "Sequence"] ("Capture mode")
                n87 = event-data() -> ()  [unwired: 1 in, 4 out]
                n88 = call <userlib>:"tm_stopcapture.vi"("error in (no error)"=w765, "Handle in"=w766) -> ("error out"=w767:errorcluster, "Handle out"=w763:u32)  [unwired: 8 in]
                n89 = call <userlib>:"tm_unpreparecapture.vi"("error in (no error)"=w767, "Handle in"=w763) -> ("error out"=w758:errorcluster, "Handle out"=w764:u32)  [unwired: 8 in]
                n90 = call <userlib>:"tm_setpropertyvalue.vi"("error in (no error)"=w758, "Value in"="Camera Readout Mode", "Property ID"=u32 4194832, "Handle in"=w764) -> ("error out"=w768:errorcluster, "Handle out"=w769:u32)  [unwired: 6 in]
                n91 = case shown="12" "Camera Readout Mode" {
                  tunnel: w769 -> [w780 w787]
                  tunnel: [w779 w782] -> w762
                  tunnel: w768 -> [w777 w792]
                  tunnel: [w776 w792] -> w760
                  frame 1, Default {
                    n92 = local read "Exposure"() -> (w778:dbl)
                    n93 = call <userlib>:"tm_setpropertyvalue.vi"("error in (no error)"=w777, "Value in"=w778, "Property ID"=u32 2031888, "Handle in"=w780) -> ("error out"=w776:errorcluster, "Handle out"=w779:u32)  [unwired: 6 in]
                  }
                  frame 12 {
                    n94 = local read "Exposure"() -> (w791:dbl)
                    n95 = local read "SVW"() -> (w789:i32)
                    n96 = formula code="slitExpos=frameInter*LW/(LinesToReadout\n+10+LW);\nlineInter = slitExpos / LW;"("frameInter"=w791, "LW"="Slit Width / Lines", "LinesToReadout"=w789) -> ("slitExpos"=w783:dbl, "lineInter"=w786:dbl)
                    n97 = call <userlib>:"tm_setpropertyvalue.vi"("Value in"=w786, "Property ID"=u32 4208720, "Handle in"=w787) -> ("Handle out"=w785:u32)  [unwired: 7 in, 1 out]
                    n98 = call <userlib>:"tm_setpropertyvalue.vi"("Value in"=w783, "Property ID"=u32 2031888, "Handle in"=w785) -> ("Handle out"=w782:u32)  [unwired: 7 in, 1 out]
                  }
                }
                n99 = call <userlib>:"tm_preparecapture.vi"("error in (no error)"=w760, "Capture mode"=w759, "Handle in"=w762) -> ("error out"=w755:errorcluster, "Buffer Info"=w761:T7, "Handle out"=w757:u32)  [unwired: 5 in, 1 out]
                n100 = call <userlib>:"tm_startcapture_b.vi"("error in (no error)"=w755, "Handle in"=w757) -> ("error out"=w754:errorcluster, "Handle out"=w756:u32)  [unwired: 8 in]
              }
              event "Ram Record": Value Change {
                n101 = event-data() -> ()  [unwired: 1 in, 5 out]
                n102 = case shown="True" "Ram Record" {
                  tunnel: w806 -> [w810 w833]
                  tunnel: w805 -> [w809 w830]
                  tunnel: [w810 w816] -> w804
                  tunnel: [w809 w818] -> w803
                  tunnel: [w808 w817] -> w799
                  tunnel: w798 -> [w808 _]
                  tunnel: w796 -> [_ w821]
                  tunnel: [_ w819] -> w795
                  tunnel: w794 -> [_ w815]
                  tunnel: w793 -> [_ w811]
                  frame False {
                  }
                  frame True {
                    w827 = 0 items=["Snap", "Sequence"] ("Capture mode")
                    # "Max 2500"
                    n103 = Flush Queue(queue=w821) -> (queue out=w820:refnum<queue>)  [unwired: 1 in, 2 out]
                    n104 = call <userlib>:"tm_stopcapture.vi"("error in (no error)"=w833, "Handle in"=w830) -> ("error out"=w832:errorcluster, "Handle out"=w831:u32)  [unwired: 8 in]
                    n105 = Bundle By Name(cluster=w811, "State"=Stack_Track."Start Sequence", "Stack Number"=0, "Image"=w815) -> (w812:T3)
                    n106 = call <userlib>:"tm_unpreparecapture.vi"("error in (no error)"=w832, "Handle in"=w831) -> ("error out"=w828:errorcluster, "Handle out"=w829:u32)  [unwired: 8 in]
                    n107 = call <userlib>:"tm_preparecapture.vi"("error in (no error)"=w828, "Frames"="Frames", "Capture mode"=w827, "Handle in"=w829) -> ("error out"=w826:errorcluster, "Buffer Info"=w824:T7, "Handle out"=w825:u32)  [unwired: 4 in, 1 out]
                    n108 = Enqueue Element(queue=w820, element=w812) -> (queue out=w822:refnum<queue>)  [unwired: 2 in, 2 out]
                    n109 = case shown="No Error" w826 {
                      selector: w826 -> [w858 w879]
                      tunnel: w825 -> [w857 w880]
                      tunnel: "Frames" -> [w853 _]
                      tunnel: [w838 w876] -> w818
                      tunnel: w824 -> [w854 _]
                      tunnel: [w837 w878] -> w816
                      tunnel: w822 -> [w852 w874]
                      tunnel: w811 -> [w851 _]
                      tunnel: [w836 w874] -> _
                      tunnel: [FALSE ("value") w888] -> w819
                      tunnel: [w835 w877] -> w817
                      frame No Error {
                        w843 = 1 items=["Snap", "Sequence"] ("Capture mode")
                        # "Frames in RAM"
                        n110 = call <userlib>:"tm_startcapture_b.vi"("error in (no error)"=w858, "Handle in"=w857) -> ("error out"=w855:errorcluster, "Handle out"=w856:u32)  [unwired: 8 in]
                        n111 = for {
                          N: w853 -> [_]
                          tunnel: w856 -> [w873]
                          tunnel: w855 -> [w872]
                          tunnel: w854 -> [w869]
                          tunnel: [w868] -> w849
                          tunnel: [w867] -> w848
                          tunnel: w852 -> [w865]
                          tunnel: Stack_Track."Collecting" ("Enum") -> [w863]
                          tunnel: w851 -> [w861]
                          tunnel: [w860] -> w842
                          i -> [w862]
                          n112 = call <userlib>:"tm_waitnextframe.vi"("error in (no error)"=w872, "Handle in"=w873) -> ("error out"=w870:errorcluster, "Frame Index"=→"Frame Index":i32, "Handle out"=w871:u32)  [unwired: 6 in, 1 out]
                          n113 = call <userlib>:"tm_getframe_a.vi"("error in (no error)"=w870, "Frame Index"=w862, "Buffer Info"=w869, "Handle in"=w871) -> ("error out"=w867:errorcluster, "Data 16"=w859:u16[][], "Handle out"=w868:u32)  [unwired: 3 in, 2 out]
                          n114 = Bundle By Name(cluster=w861, "State"=w863, "Stack Number"=w862, "Image"=w859) -> (w864:T3)
                          n115 = Enqueue Element(queue=w865, element=w864) -> (queue out=w860:refnum<queue>)  [unwired: 2 in, 2 out]
                        }
                        n116 = call <userlib>:"tm_stopcapture.vi"("error in (no error)"=w848, "Handle in"=w849) -> ("error out"=w846:errorcluster, "Handle out"=w847:u32)  [unwired: 8 in]
                        n117 = call <userlib>:"tm_unpreparecapture.vi"("error in (no error)"=w846, "Handle in"=w847) -> ("error out"=w845:errorcluster, "Handle out"=w844:u32)  [unwired: 8 in]
                        n118 = Enqueue Element(queue=w842, element=T3 {"State"=enum."End", "Stack Number"=0, "Image"=[]} ("input cluster")) -> (queue out=w836:refnum<queue>)  [unwired: 2 in, 2 out]
                        n119 = call <userlib>:"tm_preparecapture.vi"("error in (no error)"=w845, "Capture mode"=w843, "Handle in"=w844) -> ("error out"=w840:errorcluster, "Buffer Info"=w835:T7, "Handle out"=w839:u32)  [unwired: 5 in, 1 out]
                        n120 = call <userlib>:"tm_startcapture_b.vi"("error in (no error)"=w840, "Handle in"=w839) -> ("error out"=w837:errorcluster, "Handle out"=w838:u32)  [unwired: 8 in]
                      }
                      frame Error {
                        w883 = 1 items=["Snap", "Sequence"] ("Capture mode")
                        # "Prepare camera failure, likely too many frames in stack"
                        n121 = One Button Dialog(message="Too many frames in stack", button name ("OK")="OK") -> (true=w888:bool)
                        n122 = call <userlib>:"tm_stopcapture.vi"("error in (no error)"=w879, "Handle in"=w880) -> ("error out"=w886:errorcluster, "Handle out"=w887:u32)  [unwired: 8 in]
                        n123 = call <userlib>:"tm_unpreparecapture.vi"("error in (no error)"=w886, "Handle in"=w887) -> ("error out"=w885:errorcluster, "Handle out"=w884:u32)  [unwired: 8 in]
                        n124 = Enqueue Element(queue=w874, element=T3 {"State"=enum."Idle", "Stack Number"=0, "Image"=[]} ("input cluster")) -> ()  [unwired: 2 in, 3 out]
                        n125 = call <userlib>:"tm_preparecapture.vi"("error in (no error)"=w885, "Capture mode"=w883, "Handle in"=w884) -> ("error out"=w882:errorcluster, "Buffer Info"=w877:T7, "Handle out"=w881:u32)  [unwired: 5 in, 1 out]
                        n126 = call <userlib>:"tm_startcapture_b.vi"("error in (no error)"=w882, "Handle in"=w881) -> ("error out"=w878:errorcluster, "Handle out"=w876:u32)  [unwired: 8 in]
                      }
                    }
                  }
                }
              }
              event "HardDisk Record": Value Change {
                n127 = event-data() -> ()  [unwired: 1 in, 5 out]
                n128 = case shown="True" "HardDisk Record" {
                  tunnel: w903 -> [w906 w922]
                  tunnel: w902 -> [w905 w919]
                  tunnel: [w906 w909] -> w901
                  tunnel: [w905 w911] -> w900
                  tunnel: [w904 w910] -> w896
                  tunnel: w895 -> [w904 _]
                  tunnel: w893 -> [_ w907]
                  tunnel: [_ w912] -> w892
                  frame False {
                  }
                  frame True {
                    w916 = 0 items=["Snap", "Sequence"] ("Capture mode")
                    # "Max 50"
                    n129 = call <userlib>:"tm_stopcapture.vi"("error in (no error)"=w922, "Handle in"=w919) -> ("error out"=w921:errorcluster, "Handle out"=w920:u32)  [unwired: 8 in]
                    n130 = call <userlib>:"tm_unpreparecapture.vi"("error in (no error)"=w921, "Handle in"=w920) -> ("error out"=w917:errorcluster, "Handle out"=w918:u32)  [unwired: 8 in]
                    n131 = call <userlib>:"tm_preparecapture.vi"("error in (no error)"=w917, "Frames"="Frames", "Capture mode"=w916, "Handle in"=w918) -> ("error out"=w915:errorcluster, "Buffer Info"=w913:T7, "Handle out"=w914:u32)  [unwired: 4 in, 1 out]
                    n132 = case shown="No Error" w915 {
                      selector: w915 -> [w947 w960]
                      tunnel: w914 -> [w933 w961]
                      tunnel: [w936 w957] -> w911
                      tunnel: w913 -> [w944 _]
                      tunnel: [w935 w959] -> w909
                      tunnel: [FALSE ("value") w969] -> w912
                      tunnel: [w934 w958] -> w910
                      tunnel: "Frames" -> [w930 _]
                      tunnel: w907 -> [w924 w955]
                      frame No Error {
                        w939 = 1 items=["Snap", "Sequence"] ("Capture mode")
                        n133 = call <userlib>:"tm_startrecorder.vi"("frames"=w930, "File"="Temp", "Handle in"=w933) -> ("Handle out"=w932:u32)  [unwired: 7 in, 1 out]
                        n134 = call <userlib>:"tm_startcapture_b.vi"("error in (no error)"=w947, "Handle in"=w932) -> ("error out"=w945:errorcluster, "Handle out"=w946:u32)  [unwired: 8 in]
                        n135 = while {
                          tunnel: w946 -> [w953]
                          tunnel: w945 -> [w952]
                          tunnel: w944 -> [_]
                          tunnel: [w954] -> w942
                          tunnel: w930 -> [w949]
                          stop <- w950 stop-if-true
                          n136 = Wait (ms)(milliseconds to wait=u32 50) -> ()  [unwired: 1 out]
                          n137 = call <userlib>:"tm_getrecorderstatus.vi"("error in (no error)"=w952, "Handle"=w953) -> ("error out"=w954:errorcluster, "Count"=w948:i32)  [unwired: 6 in, 2 out]
                          n138 = Equal?(x=w948, y=w949) -> (x = y?=w950:bool)
                        }
                        n139 = call <userlib>:"tm_stopcapture.vi"("error in (no error)"=w942) -> ("error out"=w929:errorcluster, "Handle out"=w928:u32)  [unwired: 9 in]
                        n140 = call <userlib>:"tm_stoprecorder.vi"("error in (no error)"=w929, "Handle in"=w928) -> ("error out"=w926:errorcluster, "Handle out"=w927:u32)  [unwired: 8 in]
                        n141 = Enqueue Element(queue=w924, element=T3 {"State"=enum."Read Disk", "Stack Number"=0, "Image"=[]}, error in (no error)=w926) -> (error out=w925:errorcluster)  [unwired: 1 in, 2 out]
                        n142 = call <userlib>:"tm_unpreparecapture.vi"("error in (no error)"=w925, "Handle in"=w927) -> ("error out"=w941:errorcluster, "Handle out"=w940:u32)  [unwired: 8 in]
                        n143 = call <userlib>:"tm_preparecapture.vi"("error in (no error)"=w941, "Capture mode"=w939, "Handle in"=w940) -> ("error out"=w938:errorcluster, "Buffer Info"=w934:T7, "Handle out"=w937:u32)  [unwired: 5 in, 1 out]
                        n144 = call <userlib>:"tm_startcapture_b.vi"("error in (no error)"=w938, "Handle in"=w937) -> ("error out"=w935:errorcluster, "Handle out"=w936:u32)  [unwired: 8 in]
                      }
                      frame Error {
                        w964 = 1 items=["Snap", "Sequence"] ("Capture mode")
                        # "Prepare camera failure, likely too many frames in stack"
                        n145 = One Button Dialog(message="Too many frames in stack", button name ("OK")="OK") -> (true=w969:bool)
                        n146 = call <userlib>:"tm_stopcapture.vi"("error in (no error)"=w960, "Handle in"=w961) -> ("error out"=w967:errorcluster, "Handle out"=w968:u32)  [unwired: 8 in]
                        n147 = call <userlib>:"tm_unpreparecapture.vi"("error in (no error)"=w967, "Handle in"=w968) -> ("error out"=w966:errorcluster, "Handle out"=w965:u32)  [unwired: 8 in]
                        n148 = Enqueue Element(queue=w955, element=T3 {"State"=enum."STOP", "Stack Number"=0, "Image"=[]} ("input cluster")) -> ()  [unwired: 2 in, 3 out]
                        n149 = call <userlib>:"tm_preparecapture.vi"("error in (no error)"=w966, "Capture mode"=w964, "Handle in"=w965) -> ("error out"=w963:errorcluster, "Buffer Info"=w958:T7, "Handle out"=w962:u32)  [unwired: 5 in, 1 out]
                        n150 = call <userlib>:"tm_startcapture_b.vi"("error in (no error)"=w963, "Handle in"=w962) -> ("error out"=w959:errorcluster, "Handle out"=w957:u32)  [unwired: 8 in]
                      }
                    }
                  }
                }
              }
              event "Scan Mode": Value Change {
                w972 = u32 4211872 items=["SENSOR MODE"=4212128, "CCD MODE"=4212384, "READOUT MODE"=4211872, "ACTIVE VIEW INDEX"=4343136, "BITS PER CHANNEL"=4342976, "IMAGE PIXEL TYPE"=4343296, "BINNING"=4215968, "EXPOSURE TIME"=2049184, "CONTRAST GAIN"=3163312, "CONTRAST OFFSET"=3163328, "LIGHT MODE"=2114720, "SENSITIVITY"=2114992, "PHOTON IMAGING MODE"=2115200, "HIGH DYNAMIC RANGE MODE"=3163360, "WHITE BALANCE"=3163568, "TEMPERATURE"=2115232, "TEMPERATURE TARGET"=2115264, "SENSOR COOLER FAN"=2115296, "LINEBUNDLE HEIGHT"=4212192, "MECHANICAL SHUTTER"=2115488, "BACK FOCUS POSITION"=8422304, "TRIGGER CONNECTOR"=1066432, "TRIGGER SOURCE"=1066144, "OUTPUT TRIGGER SOURCE"=1852576, "TRIGGER GLOBAL EXPOSURE"=2049680, "FIRST TRIGGER BEHAVIOR"=2049696, "CHANNEL SYNC"=1852352, "READOUT DIRECTION"=4211904, "PRE HSYNC COUNT"=1852704] ("Parameter")
                w987 = 1 items=["Snap", "Sequence"] ("Capture mode")
                n151 = event-data() -> ("NewVal"=w977:dbl)  [unwired: 1 in, 2 out]
                n152 = call <userlib>:"tm_stopcapture.vi"("error in (no error)"=w988, "Handle in"=w989) -> ("error out"=w990:errorcluster, "Handle out"=w991:u32)  [unwired: 8 in]
                n153 = call <userlib>:"tm_unpreparecapture.vi"("error in (no error)"=w990, "Handle in"=w991) -> ("error out"=w975:errorcluster, "Handle out"=w976:u32)  [unwired: 8 in]
                n154 = call <userlib>:"tm_setparameter_a.vi"("error in (no error)"=w975, "Value in"=w977, "Parameter"=w972, "Handle in"=w976) -> ("error out"=w974:errorcluster, "Handle out"=w973:u32)  [unwired: 6 in]
                n155 = call <userlib>:"tm_getparameter_a.vi"("error in (no error)"=w974, "Parameter"=w972, "Handle in"=w973) -> ("error out"=w980:errorcluster, "Value out"=w979:dbl, "Handle out"=w978:u32)  [unwired: 6 in]
                n156 = local write "SMD"(w979) -> ()
                n157 = call <userlib>:"tm_preparecapture.vi"("error in (no error)"=w980, "Capture mode"=w987, "Handle in"=w978) -> ("error out"=w985:errorcluster, "Buffer Info"=w982:T7, "Handle out"=w986:u32)  [unwired: 5 in, 1 out]
                n158 = call <userlib>:"tm_startcapture_b.vi"("error in (no error)"=w985, "Handle in"=w986) -> ("error out"=w984:errorcluster, "Handle out"=w983:u32)  [unwired: 8 in]
              }
              event "Binning": Value Change {
                w996 = u32 4215968 items=["BINNING"=4215968, "BITS PER CHANNEL"=2, "ACTIVE VIEW INDEX"=3, "CCD MODE"=4, "SENSOR MODE"=5, "READOUT MODE"=6, "EXPOSURE TIME"=7, "CONTRAST GAIN"=8, "CONTRAST OFFSET"=9, "LIGHT MODE"=10, "SENSITIVITY"=11, "WHITE BALANCE"=12, "PHOTON IMAGING MODE"=13, "HIGH DYNAMIC RANGE MODE"=14, "TRIGGER SOURCE"=15, "TRIGGER ACTIVE"=16, "TRIGGER MODE"=17, "TRIGGER POLARITY"=18, "TRIGGER GLOBAL EXPOSURE"=19, "FIRST TRIGGER BEHAVIOR"=20, "TRIGGER TIMES"=21, "OUTPUT TRIGGER POLARITY"=22, "OUTPUT TRIGGER DELAY"=23, "OUTPUT TRIGGER PERIOD"=24, "TEMPERATURE"=25, "TEMPERATURE TARGET"=26, "SENSOR COOLER FAN"=27, "MECHANICAL SHUTTER"=28, "BACK FOCUS POSITION"=29, "FRAMEBUNDLE MODE"=30, "FRAMEBUNDLE NUMBER"=31, "LINEBUNDLE HEIGHT"=32, "TRIGGER CONNECTOR"=33, "IMAGE PIXEL TYPE"=34, "OUTPUT TRIGGER KIND"=35, "READOUT DIRECTION"=36, "CHANNEL SYNC"=37] ("Parameter")
                w1035 = 1 items=["Snap", "Sequence"] ("Capture mode")
                n159 = event-data() -> ("NewVal"=w997:u16)  [unwired: 1 in, 2 out]
                n160 = call <userlib>:"tm_stopcapture.vi"("error in (no error)"=w1004, "Handle in"=w1005) -> ("error out"=w1002:errorcluster, "Handle out"=w1003:u32)  [unwired: 8 in]
                n161 = call <userlib>:"tm_unpreparecapture.vi"("error in (no error)"=w1002, "Handle in"=w1003) -> ("error out"=w998:errorcluster, "Handle out"=w995:u32)  [unwired: 8 in]
                n162 = call <userlib>:"tm_setparameter_a.vi"("error in (no error)"=w998, "Value in"=w997, "Parameter"=w996, "Handle in"=w995) -> ("error out"=w999:errorcluster, "Handle out"=w1000:u32)  [unwired: 6 in]
                n163 = call <userlib>:"tm_getarea_a.vi"("error in (no error)"=w999, "Handle in"=w1000) -> ("error out"=w1023:errorcluster, "V Offset"=w1025:T6, "H Offset"=w1024:T6, "Handle out"=w1022:u32, "H Width"=w1026:T6, "V Width"=w1027:T6)  [unwired: 4 in]
                n164 = Unbundle By Name(w1024) -> ("Value"=w1018:i32, "Minimum"=w1021:i32, "Maximum"=w1020:i32, "Increment"=w1019:i32)
                n165 = Unbundle By Name(w1025) -> ("Value"=w1008:i32, "Minimum"=w1017:i32, "Maximum"=w1016:i32, "Increment"=w1015:i32)
                n166 = Unbundle By Name(w1026) -> ("Value"=w1007:i32, "Minimum"=w1014:i32, "Maximum"=w1013:i32, "Increment"=w1012:i32)
                n167 = Unbundle By Name(w1027) -> ("Value"=w1006:i32, "Minimum"=w1011:i32, "Maximum"=w1010:i32, "Increment"=w1009:i32)
                n168 = property on="H Offset" class="DigNum (strict)"("Value"=w1018, "Minimum"=w1021, "Maximum"=w1020, "Increment"=w1019) -> ()  [unwired: 2 in, 2 out]
                n169 = property on="V Offset" class="DigNum (strict)"("Value"=w1008, "Minimum"=w1017, "Maximum"=w1016, "Increment"=w1015) -> ()  [unwired: 2 in, 2 out]
                n170 = property on="H Width" class="DigNum (strict)"("Value"=w1007, "Minimum"=w1014, "Maximum"=w1013, "Increment"=w1012) -> ()  [unwired: 2 in, 2 out]
                n171 = property on="V Width" class="DigNum (strict)"("Value"=w1006, "Minimum"=w1011, "Maximum"=w1010, "Increment"=w1009) -> ()  [unwired: 2 in, 2 out]
                n172 = local write "SHO"(w1018) -> ()
                n173 = local write "SVO"(w1008) -> ()
                n174 = local write "SHW"(w1007) -> ()
                n175 = local write "SVW"(w1006) -> ()
                n176 = call <userlib>:"tm_preparecapture.vi"("error in (no error)"=w1023, "Capture mode"=w1035, "Handle in"=w1022) -> ("error out"=w1033:errorcluster, "Buffer Info"=w1030:T7, "Handle out"=w1034:u32)  [unwired: 5 in, 1 out]
                n177 = call <userlib>:"tm_startcapture_b.vi"("error in (no error)"=w1033, "Handle in"=w1034) -> ("error out"=w1032:errorcluster, "Handle out"=w1031:u32)  [unwired: 8 in]
              }
              event "H Offset", "H Width", "V Offset", "V Width": Value Change {
                w1080 = 1 items=["Snap", "Sequence"] ("Capture mode")
                n178 = event-data() -> ()  [unwired: 1 in, 4 out]
                n179 = call <userlib>:"tm_stopcapture.vi"("error in (no error)"=w1042, "Handle in"=w1043) -> ("error out"=w1040:errorcluster, "Handle out"=w1041:u32)  [unwired: 8 in]
                n180 = local read "H Offset"() -> (w1046:i32)
                n181 = local read "H Width"() -> (w1047:i32)
                n182 = local read "V Offset"() -> (w1048:i32)
                n183 = local read "V Width"() -> (w1045:i32)
                n184 = call <userlib>:"tm_unpreparecapture.vi"("error in (no error)"=w1040, "Handle in"=w1041) -> ("error out"=w1038:errorcluster, "Handle out"=w1039:u32)  [unwired: 8 in]
                n185 = Bundle("H Offset"=w1046, "V Offset"=w1048, "H Width"=w1047, "V Width"=w1045) -> (w1044:T8)  [unwired: 1 in]
                n186 = call <userlib>:"tm_setarea.vi"("error in (no error)"=w1038, "Sub Region"=w1044, "Handle in"=w1039) -> ("error out"=w1049:errorcluster, "Handle out"=w1050:u32)  [unwired: 7 in]
                n187 = call <userlib>:"tm_getarea_a.vi"("error in (no error)"=w1049, "Handle in"=w1050) -> ("error out"=w1068:errorcluster, "V Offset"=w1070:T6, "H Offset"=w1069:T6, "Handle out"=w1067:u32, "H Width"=w1071:T6, "V Width"=w1072:T6)  [unwired: 4 in]
                n188 = Unbundle By Name(w1069) -> ("Value"=w1063:i32, "Minimum"=w1066:i32, "Maximum"=w1065:i32, "Increment"=w1064:i32)
                n189 = Unbundle By Name(w1070) -> ("Value"=w1053:i32, "Minimum"=w1062:i32, "Maximum"=w1061:i32, "Increment"=w1060:i32)
                n190 = Unbundle By Name(w1071) -> ("Value"=w1052:i32, "Minimum"=w1059:i32, "Maximum"=w1058:i32, "Increment"=w1057:i32)
                n191 = Unbundle By Name(w1072) -> ("Value"=w1051:i32, "Minimum"=w1056:i32, "Maximum"=w1055:i32, "Increment"=w1054:i32)
                n192 = property on="H Offset" class="DigNum (strict)"("Value"=w1063, "Minimum"=w1066, "Maximum"=w1065, "Increment"=w1064) -> ()  [unwired: 2 in, 2 out]
                n193 = property on="V Offset" class="DigNum (strict)"("Value"=w1053, "Minimum"=w1062, "Maximum"=w1061, "Increment"=w1060) -> ()  [unwired: 2 in, 2 out]
                n194 = property on="H Width" class="DigNum (strict)"("Value"=w1052, "Minimum"=w1059, "Maximum"=w1058, "Increment"=w1057) -> ()  [unwired: 2 in, 2 out]
                n195 = property on="V Width" class="DigNum (strict)"("Value"=w1051, "Minimum"=w1056, "Maximum"=w1055, "Increment"=w1054) -> ()  [unwired: 2 in, 2 out]
                n196 = local write "SHO"(w1063) -> ()
                n197 = local write "SVO"(w1053) -> ()
                n198 = local write "SHW"(w1052) -> ()
                n199 = local write "SVW"(w1051) -> ()
                n200 = call <userlib>:"tm_preparecapture.vi"("error in (no error)"=w1068, "Capture mode"=w1080, "Handle in"=w1067) -> ("error out"=w1078:errorcluster, "Buffer Info"=w1075:T7, "Handle out"=w1079:u32)  [unwired: 5 in, 1 out]
                n201 = call <userlib>:"tm_startcapture_b.vi"("error in (no error)"=w1078, "Handle in"=w1079) -> ("error out"=w1077:errorcluster, "Handle out"=w1076:u32)  [unwired: 8 in]
              }
            }
            n202 = local read "stop"() -> (w584:bool)
            n203 = Unbundle By Name(w593) -> ("status"=w606:bool)
            n204 = Compound Arithmetic op=OR(w606, w584, w588) -> (w605:bool)
          }
        }
        frame Enabled {
        }
      }
      n205 = while {
        tunnel: w14 -> [w165]
        tunnel: w17 -> [w168]
        tunnel: w28 -> [w164]
        shift-right: [w163] -> _
        shift-left: w27 -> [w166]
        shift-right: [w162] -> w23
        shift-left: w26 -> [w167]
        tunnel: w25 -> [w161]
        tunnel: [w155] -> w22
        shift-right: [w153] -> _
        shift-left: _ -> [w152]
        shift-right: [w151] -> _
        shift-left: CameraControlTypeDef."Preview" ("Enum") -> [w150]
        stop <- w154 stop-if-true
        n206 = Dequeue Element(queue=w168, timeout in ms (-1)=1) -> (element=w157:T2, timed out?=w159:bool)  [unwired: 1 in, 2 out]
        n207 = case shown="True" w159 {
          tunnel: [w169 w170] -> w158
          tunnel: w157 -> [w169 _]
          tunnel: w150 -> [_ w170]
          frame False {
          }
          frame True {
          }
        }
        n208 = case shown="\"Ram Record\"" w158 {
          tunnel: w167 -> [w189 w272 w324 w367 w407 w445 w480 w484 w502 w512 w546 w567 w571]
          tunnel: w166 -> [_ _ _ _ _ w452 w474 w485 _ _ _ _ w570]
          tunnel: w165 -> [w191 w273 _ _ _ _ w479 _ _ _ _ _ _]
          tunnel: w164 -> [w192 _ _ _ _ _ w478 _ _ _ _ _ _]
          tunnel: [w176 w264 w337 w376 w414 w452 w474 w485 w488 w510 w530 w551 w570] -> w163
          tunnel: [w171 w263 w330 w374 w412 w453 w473 w484 w492 w509 w542 w563 w571] -> w162
          tunnel: w161 -> [w190 w271 w362 w402 w422 w444 w471 w483 w505 w511 w536 w557 w572]
          tunnel: [w177 w260 w336 w375 w413 w451 w472 w483 w493 w508 w541 w562 w572] -> w155
          tunnel: [w182 w266 w323 w366 w406 w443 w470 w482 w487 w507 w528 w549 w569] -> w153
          tunnel: w152 -> [w181 w266 w323 w366 w406 w443 _ w482 w487 w507 w528 w549 w569]
          tunnel: [w180 w265 w322 w365 w405 w442 CameraControlTypeDef."Preview" ("Enum") CameraControlTypeDef."Idle" ("Enum") w486 w506 w527 w548 w568] -> w151
          tunnel: w150 -> [w180 w265 w322 w365 w405 w442 _ _ w486 w506 w527 w548 w568]
          frame "Ram Record" {
            w175 = 1 items=["Snap", "Sequence"] ("Capture mode")
            n209 = call <userlib>:"tm_stopcapture.vi"("error in (no error)"=w190, "Handle in"=w189) -> ("error out"=w188:errorcluster, "Handle out"=w187:u32)  [unwired: 8 in]
            n210 = local read "Stacks"() -> (w174:dbl)
            n211 = call <userlib>:"tm_unpreparecapture.vi"("error in (no error)"=w188, "Handle in"=w187) -> ("error out"=w185:errorcluster, "Handle out"=w186:u32)  [unwired: 8 in]
            n212 = Flush Queue(queue=w191) -> (queue out=w184:refnum<queue>)  [unwired: 1 in, 2 out]
            n213 = for {
              N: w174 -> [_]
              tunnel: w192 -> [w213]
              tunnel: w184 -> [w205]
              tunnel: [w200] -> w183
              tunnel: [w199] -> w182
              tunnel: w181 -> [w198]
              shift-right: [w195] -> w172
              shift-left: w186 -> [w212]
              shift-right: [w193] -> w173
              shift-left: w185 -> [w211]
              w210 = 0 items=["Snap", "Sequence"] ("Capture mode")
              # "Max 2500"
              n214 = local read "Stack Frames"() -> (w201:i32)
              n215 = Bundle By Name(cluster=w213, "State"=Stack_Track."Start Sequence", "Stack Number"=0, "Image"=w198) -> (w202:T3)
              n216 = call <userlib>:"tm_preparecapture.vi"("error in (no error)"=w211, "Frames"=w201, "Capture mode"=w210, "Handle in"=w212) -> ("error out"=w209:errorcluster, "Buffer Info"=w207:T7, "Handle out"=w208:u32)  [unwired: 4 in, 1 out]
              n217 = Enqueue Element(queue=w205, element=w202) -> (queue out=w206:refnum<queue>)  [unwired: 2 in, 2 out]
              n218 = case shown="No Error" w209 {
                selector: w209 -> [w231 w248]
                tunnel: w208 -> [w230 w249]
                tunnel: w201 -> [w226 _]
                tunnel: [w215 w249] -> w196
                tunnel: w207 -> [w227 _]
                tunnel: [w214 w248] -> w194
                tunnel: w206 -> [w225 w251]
                tunnel: w213 -> [w224 _]
                tunnel: [w220 w251] -> _
                tunnel: [FALSE ("value") w253] -> _
                tunnel: [FALSE ("Boolean") _] -> w200
                tunnel: [w217 w250] -> w199
                tunnel: w198 -> [_ w250]
                frame No Error {
                  # "Frames in RAM"
                  n219 = call <userlib>:"tm_startcapture_b.vi"("error in (no error)"=w231, "Handle in"=w230) -> ("error out"=w228:errorcluster, "Handle out"=w229:u32)  [unwired: 8 in]
                  n220 = for {
                    N: w226 -> [_]
                    tunnel: w229 -> [w247]
                    tunnel: w228 -> [w246]
                    tunnel: w227 -> [w243]
                    tunnel: [w242] -> w215
                    tunnel: [w241] -> w214
                    tunnel: w225 -> [w240]
                    tunnel: Stack_Track."Collecting" ("Enum") -> [w238]
                    tunnel: w224 -> [w236]
                    tunnel: [w235] -> w222
                    tunnel: [w233] -> w217
                    tunnel: TRUE ("Boolean") -> [w232]
                    i -> [w237]
                    n221 = local write "Record Ready"(w232) -> ()
                    n222 = call <userlib>:"tm_waitnextframe.vi"("error in (no error)"=w246, "Handle in"=w247) -> ("error out"=w244:errorcluster, "Frame Index"=w234:i32, "Handle out"=w245:u32)  [unwired: 6 in, 1 out]
                    n223 = call <userlib>:"tm_getframe_a.vi"("error in (no error)"=w244, "Frame Index"=w237, "Buffer Info"=w243, "Handle in"=w245) -> ("error out"=w241:errorcluster, "Data 16"=w233:u16[][], "Handle out"=w242:u32)  [unwired: 3 in, 2 out]
                    n224 = Bundle By Name(cluster=w236, "State"=w238, "Stack Number"=w237, "Image"=w233) -> (w239:T3)
                    n225 = Enqueue Element(queue=w240, element=w239) -> (queue out=w235:refnum<queue>)  [unwired: 2 in, 2 out]
                    n226 = local write "Stack Frames"(w234) -> ()
                  }
                  n227 = Enqueue Element(queue=w222, element=T3 {"State"=enum."End", "Stack Number"=0, "Image"=[]} ("input cluster")) -> (queue out=w220:refnum<queue>)  [unwired: 2 in, 2 out]
                }
                frame Error {
                  # "Prepare camera failure, likely too many frames in stack"
                  n228 = One Button Dialog(message="Too many frames in stack", button name ("OK")="OK") -> (true=w253:bool)
                  n229 = Enqueue Element(queue=w251, element=T3 {"State"=enum."Idle", "Stack Number"=0, "Image"=[]} ("input cluster")) -> ()  [unwired: 2 in, 3 out]
                }
              }
              n230 = call <userlib>:"tm_stopcapture.vi"("error in (no error)"=w194, "Handle in"=w196) -> ("error out"=w197:errorcluster)  [unwired: 8 in, 1 out]
              n231 = call <userlib>:"tm_unpreparecapture.vi"("error in (no error)"=w197) -> ("error out"=w193:errorcluster, "Handle out"=w195:u32)  [unwired: 9 in]
            }
            n232 = local write "Record Ready"(w183) -> ()
            n233 = call <userlib>:"tm_preparecapture.vi"("error in (no error)"=w173, "Capture mode"=w175, "Handle in"=w172) -> ("error out"=w178:errorcluster, "Buffer Info"=w176:T7, "Handle out"=w179:u32)  [unwired: 5 in, 1 out]
            n234 = call <userlib>:"tm_startcapture_b.vi"("error in (no error)"=w178, "Handle in"=w179) -> ("error out"=w177:errorcluster, "Handle out"=w171:u32)  [unwired: 8 in]
          }
          frame "HardDisk Record" {
            w259 = 1 items=["Snap", "Sequence"] ("Capture mode")
            n235 = local read "Stacks"() -> (w256:dbl)
            n236 = call <userlib>:"tm_stopcapture.vi"("error in (no error)"=w271, "Handle in"=w272) -> ("error out"=w270:errorcluster, "Handle out"=w269:u32)  [unwired: 8 in]
            n237 = call <userlib>:"tm_unpreparecapture.vi"("error in (no error)"=w270, "Handle in"=w269) -> ("error out"=w267:errorcluster, "Handle out"=w268:u32)  [unwired: 8 in]
            n238 = for {
              N: w256 -> [_]
              tunnel: w273 -> [w284]
              shift-right: [w274] -> w257
              shift-left: w268 -> [w283]
              shift-right: [w275] -> w258
              shift-left: w267 -> [w282]
              w281 = 0 items=["Snap", "Sequence"] ("Capture mode")
              # "Would add for loop here"
              # "Max 50"
              n239 = local read "Stack Frames"() -> (w277:i32)
              n240 = call <userlib>:"tm_preparecapture.vi"("error in (no error)"=w282, "Frames"=w277, "Capture mode"=w281, "Handle in"=w283) -> ("error out"=w280:errorcluster, "Buffer Info"=w278:T7, "Handle out"=w279:u32)  [unwired: 4 in, 1 out]
              n241 = case shown="No Error" w280 {
                selector: w280 -> [w303 w315]
                tunnel: w279 -> [w297 w316]
                tunnel: w278 -> [w300 _]
                tunnel: [FALSE ("value") w319] -> _
                tunnel: w277 -> [w295 _]
                tunnel: w284 -> [w289 w313]
                tunnel: path "C:/temp.tmp" ("Temp 2") -> [w287 _]
                tunnel: [w286 w312] -> w275
                tunnel: [w285 w311] -> w274
                frame No Error {
                  n242 = call <userlib>:"tm_startrecorder.vi"("frames"=w295, "File"=w287, "Handle in"=w297) -> ("Handle out"=w296:u32)  [unwired: 7 in, 1 out]
                  n243 = call <userlib>:"tm_startcapture_b.vi"("error in (no error)"=w303, "Handle in"=w296) -> ("error out"=w301:errorcluster, "Handle out"=w302:u32)  [unwired: 8 in]
                  n244 = while {
                    tunnel: w302 -> [w309]
                    tunnel: w301 -> [w308]
                    tunnel: w300 -> [_]
                    tunnel: [w310] -> w298
                    tunnel: w295 -> [w305]
                    stop <- w306 stop-if-true
                    n245 = Wait (ms)(milliseconds to wait=u32 50) -> ()  [unwired: 1 out]
                    n246 = call <userlib>:"tm_getrecorderstatus.vi"("error in (no error)"=w308, "Handle"=w309) -> ("error out"=w310:errorcluster, "Count"=w304:i32)  [unwired: 6 in, 2 out]
                    n247 = Equal?(x=w304, y=w305) -> (x = y?=w306:bool)
                  }
                  n248 = call <userlib>:"tm_stopcapture.vi"("error in (no error)"=w298) -> ("error out"=w294:errorcluster, "Handle out"=w293:u32)  [unwired: 9 in]
                  n249 = call <userlib>:"tm_stoprecorder.vi"("error in (no error)"=w294, "Handle in"=w293) -> ("error out"=w291:errorcluster, "Handle out"=w292:u32)  [unwired: 8 in]
                  n250 = Enqueue Element(queue=w289, element=T3 {"State"=enum."Read Disk", "Stack Number"=0, "Image"=[]}, error in (no error)=w291) -> (error out=w290:errorcluster)  [unwired: 1 in, 2 out]
                  n251 = call <userlib>:"tm_unpreparecapture.vi"("error in (no error)"=w290, "Handle in"=w292) -> ("error out"=w286:errorcluster, "Handle out"=w285:u32)  [unwired: 8 in]
                }
                frame Error {
                  # "Prepare camera failure, likely too many frames in stack"
                  n252 = One Button Dialog(message="Too many frames in stack", button name ("OK")="OK") -> (true=w319:bool)
                  n253 = call <userlib>:"tm_stopcapture.vi"("error in (no error)"=w315, "Handle in"=w316) -> ("error out"=w317:errorcluster, "Handle out"=w318:u32)  [unwired: 8 in]
                  n254 = call <userlib>:"tm_unpreparecapture.vi"("error in (no error)"=w317, "Handle in"=w318) -> ("error out"=w312:errorcluster, "Handle out"=w311:u32)  [unwired: 8 in]
                  n255 = Enqueue Element(queue=w313, element=T3 {"State"=enum."STOP", "Stack Number"=0, "Image"=[]} ("input cluster")) -> ()  [unwired: 2 in, 3 out]
                }
              }
            }
            n256 = call <userlib>:"tm_preparecapture.vi"("error in (no error)"=w258, "Capture mode"=w259, "Handle in"=w257) -> ("error out"=w261:errorcluster, "Buffer Info"=w264:T7, "Handle out"=w262:u32)  [unwired: 5 in, 1 out]
            n257 = call <userlib>:"tm_startcapture_b.vi"("error in (no error)"=w261, "Handle in"=w262) -> ("error out"=w260:errorcluster, "Handle out"=w263:u32)  [unwired: 8 in]
          }
          frame "ROI" {
            w340 = 1 items=["Snap", "Sequence"] ("Capture mode")
            n258 = call <userlib>:"tm_stopcapture.vi"("error in (no error)"=w362, "Handle in"=w324) -> ("error out"=w363:errorcluster, "Handle out"=w364:u32)  [unwired: 8 in]
            n259 = call <userlib>:"tm_unpreparecapture.vi"("error in (no error)"=w363, "Handle in"=w364) -> ("error out"=w326:errorcluster, "Handle out"=w327:u32)  [unwired: 8 in]
            n260 = local read "V Width"() -> (w332:i32)
            n261 = local read "V Offset"() -> (w334:i32)
            n262 = local read "H Width"() -> (w333:i32)
            n263 = local read "H Offset"() -> (w335:i32)
            n264 = Bundle("H Offset"=w335, "V Offset"=w334, "H Width"=w333, "V Width"=w332) -> (w331:T8)  [unwired: 1 in]
            n265 = call <userlib>:"tm_setarea.vi"("error in (no error)"=w326, "Sub Region"=w331, "Handle in"=w327) -> ("error out"=w329:errorcluster, "Handle out"=w328:u32)  [unwired: 7 in]
            n266 = call <userlib>:"tm_getarea_a.vi"("error in (no error)"=w329, "Handle in"=w328) -> ("error out"=w341:errorcluster, "V Offset"=w344:T6, "H Offset"=w345:T6, "Handle out"=w325:u32, "H Width"=w343:T6, "V Width"=w342:T6)  [unwired: 4 in]
            n267 = Unbundle By Name(w345) -> ("Value"=w349:i32, "Minimum"=w346:i32, "Maximum"=w347:i32, "Increment"=w348:i32)
            n268 = Unbundle By Name(w344) -> ("Value"=w359:i32, "Minimum"=w350:i32, "Maximum"=w351:i32, "Increment"=w352:i32)
            n269 = Unbundle By Name(w343) -> ("Value"=w360:i32, "Minimum"=w353:i32, "Maximum"=w354:i32, "Increment"=w355:i32)
            n270 = Unbundle By Name(w342) -> ("Value"=w361:i32, "Minimum"=w356:i32, "Maximum"=w357:i32, "Increment"=w358:i32)
            n271 = property on="H Offset" class="DigNum (strict)"("Value"=w349, "Minimum"=w346, "Maximum"=w347, "Increment"=w348) -> ()  [unwired: 2 in, 2 out]
            n272 = property on="V Offset" class="DigNum (strict)"("Value"=w359, "Minimum"=w350, "Maximum"=w351, "Increment"=w352) -> ()  [unwired: 2 in, 2 out]
            n273 = property on="H Width" class="DigNum (strict)"("Value"=w360, "Minimum"=w353, "Maximum"=w354, "Increment"=w355) -> ()  [unwired: 2 in, 2 out]
            n274 = property on="V Width" class="DigNum (strict)"("Value"=w361, "Minimum"=w356, "Maximum"=w357, "Increment"=w358) -> ()  [unwired: 2 in, 2 out]
            n275 = local write "SHO"(w349) -> ()
            n276 = local write "SVO"(w359) -> ()
            n277 = local write "SHW"(w360) -> ()
            n278 = local write "SVW"(w361) -> ()
            n279 = call <userlib>:"tm_preparecapture.vi"("error in (no error)"=w341, "Capture mode"=w340, "Handle in"=w325) -> ("error out"=w339:errorcluster, "Buffer Info"=w337:T7, "Handle out"=w338:u32)  [unwired: 5 in, 1 out]
            n280 = call <userlib>:"tm_startcapture_b.vi"("error in (no error)"=w339, "Handle in"=w338) -> ("error out"=w336:errorcluster, "Handle out"=w330:u32)  [unwired: 8 in]
          }
          frame "Binning" {
            w379 = 1 items=["Snap", "Sequence"] ("Capture mode")
            w369 = u32 4215968 items=["BINNING"=4215968, "BITS PER CHANNEL"=2, "ACTIVE VIEW INDEX"=3, "CCD MODE"=4, "SENSOR MODE"=5, "READOUT MODE"=6, "EXPOSURE TIME"=7, "CONTRAST GAIN"=8, "CONTRAST OFFSET"=9, "LIGHT MODE"=10, "SENSITIVITY"=11, "WHITE BALANCE"=12, "PHOTON IMAGING MODE"=13, "HIGH DYNAMIC RANGE MODE"=14, "TRIGGER SOURCE"=15, "TRIGGER ACTIVE"=16, "TRIGGER MODE"=17, "TRIGGER POLARITY"=18, "TRIGGER GLOBAL EXPOSURE"=19, "FIRST TRIGGER BEHAVIOR"=20, "TRIGGER TIMES"=21, "OUTPUT TRIGGER POLARITY"=22, "OUTPUT TRIGGER DELAY"=23, "OUTPUT TRIGGER PERIOD"=24, "TEMPERATURE"=25, "TEMPERATURE TARGET"=26, "SENSOR COOLER FAN"=27, "MECHANICAL SHUTTER"=28, "BACK FOCUS POSITION"=29, "FRAMEBUNDLE MODE"=30, "FRAMEBUNDLE NUMBER"=31, "LINEBUNDLE HEIGHT"=32, "TRIGGER CONNECTOR"=33, "IMAGE PIXEL TYPE"=34, "OUTPUT TRIGGER KIND"=35, "READOUT DIRECTION"=36, "CHANNEL SYNC"=37] ("Parameter")
            n281 = local read "Binning"() -> (w401:u16)
            n282 = call <userlib>:"tm_stopcapture.vi"("error in (no error)"=w402, "Handle in"=w367) -> ("error out"=w403:errorcluster, "Handle out"=w404:u32)  [unwired: 8 in]
            n283 = call <userlib>:"tm_unpreparecapture.vi"("error in (no error)"=w403, "Handle in"=w404) -> ("error out"=w372:errorcluster, "Handle out"=w373:u32)  [unwired: 8 in]
            n284 = call <userlib>:"tm_setparameter_a.vi"("error in (no error)"=w372, "Value in"=w401, "Parameter"=w369, "Handle in"=w373) -> ("error out"=w370:errorcluster, "Handle out"=w368:u32)  [unwired: 6 in]
            n285 = call <userlib>:"tm_getarea_a.vi"("error in (no error)"=w370, "Handle in"=w368) -> ("error out"=w380:errorcluster, "V Offset"=w383:T6, "H Offset"=w384:T6, "Handle out"=w371:u32, "H Width"=w382:T6, "V Width"=w381:T6)  [unwired: 4 in]
            n286 = Unbundle By Name(w384) -> ("Value"=w388:i32, "Minimum"=w385:i32, "Maximum"=w386:i32, "Increment"=w387:i32)
            n287 = Unbundle By Name(w383) -> ("Value"=w398:i32, "Minimum"=w389:i32, "Maximum"=w390:i32, "Increment"=w391:i32)
            n288 = Unbundle By Name(w382) -> ("Value"=w399:i32, "Minimum"=w392:i32, "Maximum"=w393:i32, "Increment"=w394:i32)
            n289 = Unbundle By Name(w381) -> ("Value"=w400:i32, "Minimum"=w395:i32, "Maximum"=w396:i32, "Increment"=w397:i32)
            n290 = property on="H Offset" class="DigNum (strict)"("Value"=w388, "Minimum"=w385, "Maximum"=w386, "Increment"=w387) -> ()  [unwired: 2 in, 2 out]
            n291 = property on="V Offset" class="DigNum (strict)"("Value"=w398, "Minimum"=w389, "Maximum"=w390, "Increment"=w391) -> ()  [unwired: 2 in, 2 out]
            n292 = property on="H Width" class="DigNum (strict)"("Value"=w399, "Minimum"=w392, "Maximum"=w393, "Increment"=w394) -> ()  [unwired: 2 in, 2 out]
            n293 = property on="V Width" class="DigNum (strict)"("Value"=w400, "Minimum"=w395, "Maximum"=w396, "Increment"=w397) -> ()  [unwired: 2 in, 2 out]
            n294 = local write "SHO"(w388) -> ()
            n295 = local write "SVO"(w398) -> ()
            n296 = local write "SHW"(w399) -> ()
            n297 = local write "SVW"(w400) -> ()
            n298 = call <userlib>:"tm_preparecapture.vi"("error in (no error)"=w380, "Capture mode"=w379, "Handle in"=w371) -> ("error out"=w378:errorcluster, "Buffer Info"=w376:T7, "Handle out"=w377:u32)  [unwired: 5 in, 1 out]
            n299 = call <userlib>:"tm_startcapture_b.vi"("error in (no error)"=w378, "Handle in"=w377) -> ("error out"=w375:errorcluster, "Handle out"=w374:u32)  [unwired: 8 in]
          }
          frame "Readout Mode" {
            w417 = 1 items=["Snap", "Sequence"] ("Capture mode")
            n300 = call <userlib>:"tm_stopcapture.vi"("error in (no error)"=w422, "Handle in"=w407) -> ("error out"=w423:errorcluster, "Handle out"=w424:u32)  [unwired: 8 in]
            n301 = call <userlib>:"tm_unpreparecapture.vi"("error in (no error)"=w423, "Handle in"=w424) -> ("error out"=w408:errorcluster, "Handle out"=w409:u32)  [unwired: 8 in]
            n302 = local read "Camera Readout Mode"() -> (w420:u16)
            n303 = call <userlib>:"tm_setpropertyvalue.vi"("error in (no error)"=w408, "Value in"=w420, "Property ID"=u32 4194832, "Handle in"=w409) -> ("error out"=w418:errorcluster, "Handle out"=w419:u32)  [unwired: 6 in]
            n304 = case shown="12" w420 {
              tunnel: [w428 w433] -> w411
              tunnel: w419 -> [w427 w434]
              tunnel: w418 -> [w426 w433]
              tunnel: [w425 w432] -> w410
              frame 1, Default {
                n305 = local read "Exposure"() -> (w429:dbl)
                n306 = call <userlib>:"tm_setpropertyvalue.vi"("error in (no error)"=w426, "Value in"=w429, "Property ID"=u32 2031888, "Handle in"=w427) -> ("error out"=w428:errorcluster, "Handle out"=w425:u32)  [unwired: 6 in]
              }
              frame 12 {
                n307 = local read "Slit Width / Lines"() -> (w431:sgl)
                n308 = local read "Exposure"() -> (w441:dbl)
                n309 = local read "SVW"() -> (w440:i32)
                n310 = formula code="slitExpos=frameInter*LW/(LinesToReadout\n+10+LW);\nlineInter = slitExpos / LW;"("frameInter"=w441, "LW"=w431, "LinesToReadout"=w440) -> ("slitExpos"=w435:dbl, "lineInter"=w438:dbl)
                n311 = call <userlib>:"tm_setpropertyvalue.vi"("Value in"=w438, "Property ID"=u32 4208720, "Handle in"=w434) -> ("Handle out"=w437:u32)  [unwired: 7 in, 1 out]
                n312 = call <userlib>:"tm_setpropertyvalue.vi"("Value in"=w435, "Property ID"=u32 2031888, "Handle in"=w437) -> ("Handle out"=w432:u32)  [unwired: 7 in, 1 out]
              }
            }
            n313 = call <userlib>:"tm_preparecapture.vi"("error in (no error)"=w411, "Capture mode"=w417, "Handle in"=w410) -> ("error out"=w416:errorcluster, "Buffer Info"=w414:T7, "Handle out"=w415:u32)  [unwired: 5 in, 1 out]
            n314 = call <userlib>:"tm_startcapture_b.vi"("error in (no error)"=w416, "Handle in"=w415) -> ("error out"=w413:errorcluster, "Handle out"=w412:u32)  [unwired: 8 in]
          }
          frame "Update" {
            w449 = u32 1066144 items=["SENSOR MODE"=4212128, "CCD MODE"=4212384, "READOUT MODE"=4211872, "ACTIVE VIEW INDEX"=4343136, "BITS PER CHANNEL"=4342976, "IMAGE PIXEL TYPE"=4343296, "BINNING"=4215968, "EXPOSURE TIME"=2049184, "CONTRAST GAIN"=3163312, "CONTRAST OFFSET"=3163328, "LIGHT MODE"=2114720, "SENSITIVITY"=2114992, "PHOTON IMAGING MODE"=2115200, "HIGH DYNAMIC RANGE MODE"=3163360, "WHITE BALANCE"=3163568, "TEMPERATURE"=2115232, "TEMPERATURE TARGET"=2115264, "SENSOR COOLER FAN"=2115296, "LINEBUNDLE HEIGHT"=4212192, "MECHANICAL SHUTTER"=2115488, "BACK FOCUS POSITION"=8422304, "TRIGGER CONNECTOR"=1066432, "TRIGGER SOURCE"=1066144, "OUTPUT TRIGGER SOURCE"=1852576, "TRIGGER GLOBAL EXPOSURE"=2049680, "FIRST TRIGGER BEHAVIOR"=2049696, "CHANNEL SYNC"=1852352, "READOUT DIRECTION"=4211904, "PRE HSYNC COUNT"=1852704] ("Parameter")
            w454 = u32 2049184 items=["SENSOR MODE"=4212128, "CCD MODE"=4212384, "READOUT MODE"=4211872, "ACTIVE VIEW INDEX"=4343136, "BITS PER CHANNEL"=4342976, "IMAGE PIXEL TYPE"=4343296, "BINNING"=4215968, "EXPOSURE TIME"=2049184, "CONTRAST GAIN"=3163312, "CONTRAST OFFSET"=3163328, "LIGHT MODE"=2114720, "SENSITIVITY"=2114992, "PHOTON IMAGING MODE"=2115200, "HIGH DYNAMIC RANGE MODE"=3163360, "WHITE BALANCE"=3163568, "TEMPERATURE"=2115232, "TEMPERATURE TARGET"=2115264, "SENSOR COOLER FAN"=2115296, "LINEBUNDLE HEIGHT"=4212192, "MECHANICAL SHUTTER"=2115488, "BACK FOCUS POSITION"=8422304, "TRIGGER CONNECTOR"=1066432, "TRIGGER SOURCE"=1066144, "OUTPUT TRIGGER SOURCE"=1852576, "TRIGGER GLOBAL EXPOSURE"=2049680, "FIRST TRIGGER BEHAVIOR"=2049696, "CHANNEL SYNC"=1852352, "READOUT DIRECTION"=4211904, "PRE HSYNC COUNT"=1852704] ("Parameter")
            # "Fails"
            # "Error on get"
            n315 = local read "Exposure"() -> (w456:dbl)
            n316 = disable-structure shown="Disabled" {
              disable-tunnel: w445 -> [w461 _]
              disable-tunnel: w444 -> [w460 _]
              frame Disabled {
                w459 = u32 4226016 items=["SENSOR MODE"=4212128, "CCD MODE"=4212384, "READOUT MODE"=4211872, "ACTIVE VIEW INDEX"=4343136, "BITS PER CHANNEL"=4342976, "IMAGE PIXEL TYPE"=4343296, "BINNING"=4215968, "EXPOSURE TIME"=2049184, "CONTRAST GAIN"=3163312, "CONTRAST OFFSET"=3163328, "LIGHT MODE"=2114720, "SENSITIVITY"=2114992, "PHOTON IMAGING MODE"=2115200, "HIGH DYNAMIC RANGE MODE"=3163360, "WHITE BALANCE"=3163568, "TEMPERATURE"=2115232, "TEMPERATURE TARGET"=2115264, "SENSOR COOLER FAN"=2115296, "LINEBUNDLE HEIGHT"=4212192, "MECHANICAL SHUTTER"=2115488, "BACK FOCUS POSITION"=8422304, "TRIGGER CONNECTOR"=1066432, "TRIGGER SOURCE"=1066144, "OUTPUT TRIGGER SOURCE"=1852576, "TRIGGER GLOBAL EXPOSURE"=2049680, "FIRST TRIGGER BEHAVIOR"=2049696, "CHANNEL SYNC"=1852352, "READOUT DIRECTION"=4211904, "PRE HSYNC COUNT"=1852704, "INTERNAL LINE SPEED"=4226000, "INTERNAL LINE INTERVAL"=4226016] ("Parameter")
                n317 = local read "Internal Line Interval"() -> (w463:dbl)
                n318 = call <userlib>:"tm_setparameter_a.vi"("error in (no error)"=w460, "Value in"=w463, "Parameter"=w459, "Handle in"=w461) -> ("error out"=w462:errorcluster, "Handle out"=w465:u32)  [unwired: 6 in]
                n319 = call <userlib>:"tm_getparameter_a.vi"("error in (no error)"=w462, "Parameter"=w459, "Handle in"=w465) -> ("Value out"=w464:dbl)  [unwired: 6 in, 2 out]
                n320 = local write "Internal Line Interval"(w464) -> ()
              }
              frame Enabled {
              }
            }
            n321 = call <userlib>:"tm_setparameter_a.vi"("error in (no error)"=w444, "Value in"=w456, "Parameter"=w454, "Handle in"=w445) -> ("error out"=w458:errorcluster, "Handle out"=w455:u32)  [unwired: 6 in]
            n322 = call <userlib>:"tm_getparameter_a.vi"("error in (no error)"=w458, "Parameter"=w454, "Handle in"=w455) -> ("Value out"=w457:dbl)  [unwired: 6 in, 2 out]
            n323 = local write "EXP"(w457) -> ()
            n324 = local read "Trigger Source"() -> (w447:sgl)
            n325 = call <userlib>:"tm_setparameter_a.vi"("error in (no error)"=w444, "Value in"=w447, "Parameter"=w449, "Handle in"=w445) -> ("error out"=w446:errorcluster, "Handle out"=w450:u32)  [unwired: 6 in]
            n326 = call <userlib>:"tm_getparameter_a.vi"("error in (no error)"=w446, "Parameter"=w449, "Handle in"=w450) -> ("error out"=w451:errorcluster, "Value out"=w448:dbl, "Handle out"=w453:u32)  [unwired: 6 in]
            n327 = local write "Trigger Source"(w448) -> ()
          }
          frame "Preview", Default {
            # "Slows it all down somewhat"
            # "Currently the external trigger setting means that frames are dropped because the system lingers at this point. \nIdeally I should set it so when the system is external and recording it won't run this section.\n\nThis is what HC Image does, it offers no live video when you switch from live to record mode.\n\nRealistically when tirgger set external and this times out once then ignore this step.\nBut it'd have to be reset after a recording.\n\nNeed to think more betterer about how to handle this else frames will just be dropped. Probably best to just have a seperate scan mode\nOr at least just a boolean to turn off this live capture section. Working now maybe"
            n328 = call <userlib>:"tm_waitnextframe.vi"("error in (no error)"=w471, "Timeout"=3000, "Handle in"=w480) -> ("error out"=w467:errorcluster, "Handle out"=w468:u32)  [unwired: 5 in, 2 out]
            n329 = call <userlib>:"tm_getframe_a.vi"("error in (no error)"=w467, "Buffer Info"=w474, "Handle in"=w468) -> ("error out"=w472:errorcluster, "Data 16"=w470:u16[][], "Handle out"=w473:u32)  [unwired: 4 in, 2 out]
            n330 = Bundle By Name(cluster=w478, "State"=Stack_Track."Idle", "Stack Number"=0, "Image"=w470) -> (w475:T3)
            n331 = Enqueue Element(queue=w479, element=w475) -> ()  [unwired: 2 in, 3 out]
          }
          frame "Idle" {
          }
          frame "Scan Mode" {
            w489 = 1 items=["Snap", "Sequence"] ("Capture mode")
            w498 = u32 4211872 items=["SENSOR MODE"=4212128, "CCD MODE"=4212384, "READOUT MODE"=4211872, "ACTIVE VIEW INDEX"=4343136, "BITS PER CHANNEL"=4342976, "IMAGE PIXEL TYPE"=4343296, "BINNING"=4215968, "EXPOSURE TIME"=2049184, "CONTRAST GAIN"=3163312, "CONTRAST OFFSET"=3163328, "LIGHT MODE"=2114720, "SENSITIVITY"=2114992, "PHOTON IMAGING MODE"=2115200, "HIGH DYNAMIC RANGE MODE"=3163360, "WHITE BALANCE"=3163568, "TEMPERATURE"=2115232, "TEMPERATURE TARGET"=2115264, "SENSOR COOLER FAN"=2115296, "LINEBUNDLE HEIGHT"=4212192, "MECHANICAL SHUTTER"=2115488, "BACK FOCUS POSITION"=8422304, "TRIGGER CONNECTOR"=1066432, "TRIGGER SOURCE"=1066144, "OUTPUT TRIGGER SOURCE"=1852576, "TRIGGER GLOBAL EXPOSURE"=2049680, "FIRST TRIGGER BEHAVIOR"=2049696, "CHANNEL SYNC"=1852352, "READOUT DIRECTION"=4211904, "PRE HSYNC COUNT"=1852704] ("Parameter")
            n332 = call <userlib>:"tm_stopcapture.vi"("error in (no error)"=w505, "Handle in"=w502) -> ("error out"=w504:errorcluster, "Handle out"=w503:u32)  [unwired: 8 in]
            n333 = call <userlib>:"tm_unpreparecapture.vi"("error in (no error)"=w504, "Handle in"=w503) -> ("error out"=w500:errorcluster, "Handle out"=w501:u32)  [unwired: 8 in]
            n334 = local read "Scan Mode"() -> (w499:dbl)
            n335 = call <userlib>:"tm_setparameter_a.vi"("error in (no error)"=w500, "Value in"=w499, "Parameter"=w498, "Handle in"=w501) -> ("error out"=w494:errorcluster)  [unwired: 6 in, 1 out]
            n336 = call <userlib>:"tm_getparameter_a.vi"("error in (no error)"=w494, "Parameter"=w498) -> ("error out"=w495:errorcluster, "Value out"=w497:dbl, "Handle out"=w490:u32)  [unwired: 7 in]
            n337 = local write "SMD"(w497) -> ()
            n338 = call <userlib>:"tm_preparecapture.vi"("error in (no error)"=w495, "Capture mode"=w489, "Handle in"=w490) -> ("error out"=w496:errorcluster, "Buffer Info"=w488:T7, "Handle out"=w491:u32)  [unwired: 5 in, 1 out]
            n339 = call <userlib>:"tm_startcapture_b.vi"("error in (no error)"=w496, "Handle in"=w491) -> ("error out"=w493:errorcluster, "Handle out"=w492:u32)  [unwired: 8 in]
          }
          frame "Trigger Mode" {
            w513 = u32 1049104 ("Property ID")
            n340 = local read "Trigger Mode"() -> (w518:sgl)
            n341 = call <userlib>:"tm_stopcapture.vi"("error in (no error)"=w511, "Handle in"=w512) -> ("error out"=w517:errorcluster, "Handle out"=w525:u32)  [unwired: 8 in]
            n342 = call <userlib>:"tm_unpreparecapture.vi"("error in (no error)"=w517, "Handle in"=w525) -> ("error out"=w515:errorcluster, "Handle out"=w521:u32)  [unwired: 8 in]
            n343 = call <userlib>:"tm_setpropertyvalue.vi"("error in (no error)"=w515, "Value in"=w518, "Property ID"=w513, "Handle in"=w521) -> ("error out"=w514:errorcluster, "Handle out"=w520:u32)  [unwired: 6 in]
            n344 = call <userlib>:"tm_getpropertyvalue.vi"("error in (no error)"=w514, "Property ID"=w513, "Handle in"=w520) -> ("error out"=w522:errorcluster, "Value in"=w519:sgl, "Handle out"=w523:u32)  [unwired: 6 in]
            n345 = local write "Trigger Mode"(w519) -> ()
            n346 = call <userlib>:"tm_preparecapture.vi"("error in (no error)"=w522, "Handle in"=w523) -> ("error out"=w516:errorcluster, "Buffer Info"=w510:T7, "Handle out"=w524:u32)  [unwired: 6 in, 1 out]
            n347 = call <userlib>:"tm_startcapture_b.vi"("error in (no error)"=w516, "Handle in"=w524) -> ("error out"=w508:errorcluster, "Handle out"=w509:u32)  [unwired: 8 in]
          }
          frame "Readout Direction" {
            w526 = u32 4211904 items=["SENSOR MODE"=4212128, "CCD MODE"=4212384, "READOUT MODE"=4211872, "ACTIVE VIEW INDEX"=4343136, "BITS PER CHANNEL"=4342976, "IMAGE PIXEL TYPE"=4343296, "BINNING"=4215968, "EXPOSURE TIME"=2049184, "CONTRAST GAIN"=3163312, "CONTRAST OFFSET"=3163328, "LIGHT MODE"=2114720, "SENSITIVITY"=2114992, "PHOTON IMAGING MODE"=2115200, "HIGH DYNAMIC RANGE MODE"=3163360, "WHITE BALANCE"=3163568, "TEMPERATURE"=2115232, "TEMPERATURE TARGET"=2115264, "SENSOR COOLER FAN"=2115296, "LINEBUNDLE HEIGHT"=4212192, "MECHANICAL SHUTTER"=2115488, "BACK FOCUS POSITION"=8422304, "TRIGGER CONNECTOR"=1066432, "TRIGGER SOURCE"=1066144, "OUTPUT TRIGGER SOURCE"=1852576, "TRIGGER GLOBAL EXPOSURE"=2049680, "FIRST TRIGGER BEHAVIOR"=2049696, "CHANNEL SYNC"=1852352, "READOUT DIRECTION"=4211904, "PRE HSYNC COUNT"=1852704, "INTERNAL LINE SPEED"=4226000, "INTERNAL LINE INTERVAL"=4226016] ("Parameter")
            w537 = 1 items=["Snap", "Sequence"] ("Capture mode")
            n348 = call <userlib>:"tm_stopcapture.vi"("error in (no error)"=w536, "Handle in"=w546) -> ("error out"=w538:errorcluster, "Handle out"=w545:u32)  [unwired: 8 in]
            n349 = call <userlib>:"tm_unpreparecapture.vi"("error in (no error)"=w538, "Handle in"=w545) -> ("error out"=w539:errorcluster, "Handle out"=w544:u32)  [unwired: 8 in]
            n350 = local read "Readout Direction"() -> (w529:sgl)
            n351 = call <userlib>:"tm_setparameter_a.vi"("error in (no error)"=w539, "Value in"=w529, "Parameter"=w526, "Handle in"=w544) -> ("error out"=w533:errorcluster, "Handle out"=w535:u32)  [unwired: 6 in]
            n352 = call <userlib>:"tm_getparameter_a.vi"("error in (no error)"=w533, "Parameter"=w526, "Handle in"=w535) -> ("error out"=w532:errorcluster, "Value out"=w531:dbl, "Handle out"=w534:u32)  [unwired: 6 in]
            n353 = local write "Readout Direction"(w531) -> ()
            n354 = call <userlib>:"tm_preparecapture.vi"("error in (no error)"=w532, "Capture mode"=w537, "Handle in"=w534) -> ("error out"=w540:errorcluster, "Buffer Info"=w530:T7, "Handle out"=w543:u32)  [unwired: 5 in, 1 out]
            n355 = call <userlib>:"tm_startcapture_b.vi"("error in (no error)"=w540, "Handle in"=w543) -> ("error out"=w541:errorcluster, "Handle out"=w542:u32)  [unwired: 8 in]
          }
          frame "IntervalLineInt" {
            w547 = 4226016
            w558 = 1 items=["Snap", "Sequence"] ("Capture mode")
            n356 = call <userlib>:"tm_stopcapture.vi"("error in (no error)"=w557, "Handle in"=w567) -> ("error out"=w559:errorcluster, "Handle out"=w566:u32)  [unwired: 8 in]
            n357 = call <userlib>:"tm_unpreparecapture.vi"("error in (no error)"=w559, "Handle in"=w566) -> ("error out"=w560:errorcluster, "Handle out"=w565:u32)  [unwired: 8 in]
            n358 = local read "Internal Line Interval"() -> (w550:dbl)
            n359 = call <userlib>:"tm_setparameter_a.vi"("error in (no error)"=w560, "Value in"=w550, "Parameter"=w547, "Handle in"=w565) -> ("error out"=w554:errorcluster, "Handle out"=w556:u32)  [unwired: 6 in]
            n360 = call <userlib>:"tm_getparameter_a.vi"("error in (no error)"=w554, "Parameter"=w547, "Handle in"=w556) -> ("error out"=w553:errorcluster, "Value out"=w552:dbl, "Handle out"=w555:u32)  [unwired: 6 in]
            n361 = local write "Internal Line Interval"(w552) -> ()
            n362 = call <userlib>:"tm_preparecapture.vi"("error in (no error)"=w553, "Capture mode"=w558, "Handle in"=w555) -> ("error out"=w561:errorcluster, "Buffer Info"=w551:T7, "Handle out"=w564:u32)  [unwired: 5 in, 1 out]
            n363 = call <userlib>:"tm_startcapture_b.vi"("error in (no error)"=w561, "Handle in"=w564) -> ("error out"=w562:errorcluster, "Handle out"=w563:u32)  [unwired: 8 in]
          }
          frame "Disengage Update" {
          }
        }
        n364 = local read "stop"() -> (w156:bool)
        n365 = Compound Arithmetic op=OR(w156, w155) -> (w154:bool)
      }
      n366 = while {
        tunnel: w14 -> [w1097]
        shift-right: [w1093] -> _
        shift-left: _ -> [w1091]
        shift-right: [w1090] -> _
        shift-left: w9 -> [w1083]
        shift-right: [w1088] -> _
        shift-left: _ -> [w1084]
        stop <- w1092 stop-if-true
        n367 = Dequeue Element(queue=w1097, error in (no error)=w1083) -> (element=w1096:T3, timed out?=w1085:bool, error out=w1082:errorcluster)  [unwired: 1 in, 1 out]
        n368 = Unbundle By Name(w1096) -> ("State"=w1095:T1, "Stack Number"=w1094:i32, "Image"=w1086:u16[][])
        "State" <- w1095
        n369 = case shown="False" w1085 {
          tunnel: w1086 -> [w1099 w1101]
          tunnel: [w1099 w1100] -> w1087
          tunnel: [w1098 w1101] -> w1088
          tunnel: w1084 -> [w1098 w1100]
          frame False {
          }
          frame True {
          }
        }
        "Image" <- w1087
        n370 = case shown="\"Read Disk\"" w1095 {
          tunnel: w1094 -> [_ _ _ _ _ _]
          tunnel: [w1104 w1121 _ _ _ _] -> w1093
          tunnel: w1091 -> [_ w1122 w1128 _ _ _]
          tunnel: [FALSE _ _ _ TRUE _] -> w1092
          tunnel: w1087 -> [w1102 w1123 _ _ _ _]
          tunnel: w1082 -> [_ w1120 w1126 w1138 w1163 w1165]
          tunnel: [w1105 w1119 w1127 w1135 w1163 w1165] -> w1090
          tunnel: "Path" -> [w1108 _ _ w1140 _ _]
          frame "Start Sequence" {
            # "Public tiff library"
            # "Get path and open file"
            n371 = Equal?(x=w1108, y=path "") -> (x = y?=w1110:bool)
            n372 = case shown="True" w1110 {
              tunnel: w1108 -> [w1112 _]
              tunnel: [w1112 w1115] -> w1107
              frame False {
              }
              frame True {
                n373 = call "File Dialog"("pattern (all files)"=".tiff", "pattern label"="Tiff Image") -> ("selected path"=w1115:path)  [unwired: 10 in, 3 out]
              }
            }
            n374 = case shown="True" "AutoIncrement" {
              tunnel: w1107 -> [w1116 w1118]
              tunnel: [w1116 w1117] -> w1103
              frame False {
              }
              frame True {
                n375 = call "4Digit File Incrementer.vi"("path"=w1118) -> ("appended path"=w1117:path)  [unwired: 10 in]
              }
            }
            n376 = local write "Path"(w1103) -> ()
            n377 = call-poly "CTIFFNewFileAndStyle.vi"("image"=w1102, "output_file"=w1103) -> ("error"=w1105:errorcluster, "CTIFF"=w1104:i64)  [unwired: 8 in]
          }
          frame "Collecting" {
            # "Add Image to write scan line"
            n378 = call-poly "CTIFFAddNewPage.vi"("error"=w1120, "image"=w1123, "CTIFF"=w1122) -> ("error"=w1119:errorcluster, "CTIFF"=w1121:i64)  [unwired: 7 in]
            n379 = property on="Ram Record" class="Bool (strict)"("DisabledEnum"=T4."Disabled and Grayed Out" ("Disabled"), "BoolText.Text"="Saving" ("Boolean Text.Text")) -> ()  [unwired: 2 in, 2 out]
          }
          frame "End" {
            (unwired) FALSE
            # "Close image file, reset capturing button"
            n380 = call "CTIFFWriteAndClose.vi"("error"=w1126, "CTIFF"=w1128) -> ("error"=w1127:errorcluster)  [unwired: 9 in]
            n381 = property on="Ram Record" class="Bool (strict)"("BoolText.Text"="RAM" ("Boolean Text.Text"), "DisabledEnum"=T4."Enabled" ("Disabled")) -> ()  [unwired: 2 in, 2 out]
          }
          frame "Read Disk" {
            w1131 = path "C:/temp.tmp" ("Temp 2")
            # "Can't just send hardisk record in a loop a bunch of times though.\nHave to modify consumer"
            # "This is the easiest option."
            # "Could potentially implments stacks into ram and hardisk record"
            # "For instance the harddisk record may be set to record 5000 images, this could then be used to chunk that into\n50 stacks of 100"
            # "Use stacks one day for rapid imaging , whatevr."
            n382 = call <userlib>:"tm_opendcimgfile.vi"("Path"=w1131) -> ("Total Frames"=w1141:i32, "File Handle"=w1142:u32)  [unwired: 8 in, 1 out]
            n383 = for {
              N: w1141 -> [_]
              tunnel: w1140 -> [w1150]
              shift-right: [w1148] -> w1136
              shift-left: i64 0 ("CTIFF") -> [w1149]
              tunnel: [w1147] -> w1137
              tunnel: w1138 -> [w1146]
              shift-right: [w1152] -> w1132
              shift-left: w1142 -> [w1153]
              i -> [w1143]
              n384 = local write "Stack Frames"(w1143) -> ()
              n385 = Equal To 0?(x=w1143) -> (x = 0?=w1151:bool)
              n386 = call <userlib>:"tm_getdcimgframe.vi"("error in (no error)"=w1146, "Frame Index"=w1143, "File Handle in"=w1153) -> ("error out"=w1145:errorcluster, "Data"=w1144:u16[][], "File Handle out"=w1152:u32)  [unwired: 5 in, 1 out]
              n387 = local write "Image"(w1144) -> ()
              n388 = case shown="True" w1151 {
                tunnel: w1150 -> [_ w1162]
                tunnel: w1144 -> [w1154 w1161]
                tunnel: w1149 -> [w1158 _]
                tunnel: [w1157 w1160] -> w1148
                tunnel: [w1156 w1159] -> w1147
                tunnel: w1145 -> [w1155 _]
                frame False {
                  n389 = call-poly "CTIFFAddNewPage.vi"("error"=w1155, "image"=w1154, "CTIFF"=w1158) -> ("error"=w1156:errorcluster, "CTIFF"=w1157:i64)  [unwired: 7 in]
                }
                frame True {
                  n390 = call-poly "CTIFFNewFileAndStyle.vi"("image"=w1161, "output_file"=w1162) -> ("error"=w1159:errorcluster, "CTIFF"=w1160:i64)  [unwired: 8 in]
                }
              }
            }
            n391 = call "CTIFFWriteAndClose.vi"("error"=w1137, "CTIFF"=w1136) -> ("error"=w1134:errorcluster)  [unwired: 9 in]
            n392 = call <userlib>:"tm_closedcimgfile.vi"("error in (no error)"=w1134, "File Handle"=w1132) -> ("error out"=w1133:errorcluster)  [unwired: 9 in]
            n393 = Delete(path (use dialog)=w1131, error in=w1133) -> (error out=w1135:errorcluster)  [unwired: 3 in, 2 out]
          }
          frame "STOP" {
          }
          frame "Idle" {
          }
        }
      }
      n394 = while {
        tunnel: w17 -> [w100]
        stop <- "stop" stop-if-true
        n395 = event shown="[8] \"HardDisk Record\": Value Change" {
          selector: _ -> [_ _ _ _ _ _ _ _ _ _ _ _ _]
          dyn-events: _ -> [_ _ _ _ _ _ _ _ _ _ _ _ _]
          timeout: _ -> [_ _ _ _ _ _ _ _ _ _ _ _ _]
          tunnel: w100 -> [_ w102 w104 w105 w107 w110 w113 w117 w122 w125 w129 w139 w149]
          event Timeout {
            n396 = event-data() -> ()  [unwired: 1 in, 3 out]
          }
          event "Camera Readout Mode": Value Change {
            n397 = event-data() -> ()  [unwired: 1 in, 6 out]
            n398 = Enqueue Element(queue=w102, element=CameraControlTypeDef."Readout Mode" ("Enum")) -> ()  [unwired: 2 in, 3 out]
          }
          event "V Width", "V Offset", "H Width", "H Offset": Value Change {
            n399 = event-data() -> ()  [unwired: 1 in, 6 out]
            n400 = Enqueue Element(queue=w104, element=CameraControlTypeDef."ROI" ("Enum")) -> ()  [unwired: 2 in, 3 out]
          }
          event "Readout Direction": Value Change {
            n401 = event-data() -> ()  [unwired: 1 in, 6 out]
            n402 = Enqueue Element(queue=w105, element=CameraControlTypeDef."Readout Direction" ("Enum")) -> ()  [unwired: 2 in, 3 out]
          }
          event "Binning": Value Change {
            n403 = event-data() -> ()  [unwired: 1 in, 6 out]
            n404 = Enqueue Element(queue=w107, element=CameraControlTypeDef."Binning" ("Enum")) -> ()  [unwired: 2 in, 3 out]
          }
          event "Ram Record": Value Change {
            n405 = event-data() -> ("NewVal"=w109:bool)  [unwired: 1 in, 5 out]
            n406 = case shown="True" w109 {
              tunnel: w110 -> [_ w111]
              frame False {
              }
              frame True {
                n407 = Enqueue Element(queue=w111, element=CameraControlTypeDef."Ram Record" ("Enum")) -> ()  [unwired: 2 in, 3 out]
              }
            }
          }
          event "Capture Mode": Value Change {
            n408 = event-data() -> ("NewVal"=w114:bool)  [unwired: 1 in, 5 out]
            n409 = case shown="True" w114 {
              tunnel: w113 -> [_ w116]
              frame False {
              }
              frame True {
                n410 = Enqueue Element(queue=w116, element=CameraControlTypeDef."Idle") -> ()  [unwired: 2 in, 3 out]
              }
            }
          }
          event "Preview": Value Change {
            n411 = event-data() -> ("NewVal"=w118:bool)  [unwired: 1 in, 5 out]
            n412 = case shown="True" w118 {
              tunnel: w117 -> [_ w120]
              frame False {
              }
              frame True {
                n413 = Enqueue Element(queue=w120, element=CameraControlTypeDef."Preview") -> ()  [unwired: 2 in, 3 out]
              }
            }
          }
          event "HardDisk Record": Value Change {
            n414 = event-data() -> ("NewVal"=w121:bool)  [unwired: 1 in, 5 out]
            n415 = case shown="True" w121 {
              tunnel: w122 -> [_ w123]
              frame False {
              }
              frame True {
                n416 = Enqueue Element(queue=w123, element=CameraControlTypeDef."HardDisk Record" ("Enum")) -> ()  [unwired: 2 in, 3 out]
              }
            }
          }
          event "Exposure": Value Change {
            n417 = event-data() -> ()  [unwired: 1 in, 6 out]
            n418 = Enqueue Element(queue=w125, element=CameraControlTypeDef."Update" ("Enum")) -> ()  [unwired: 2 in, 3 out]
          }
          event "Trigger Source": Value Change {
            n419 = event-data() -> ("NewVal"=w127:sgl)  [unwired: 1 in, 5 out]
            n420 = case shown="1, Default" w127 {
              tunnel: w129 -> [w132 w135]
              tunnel: [w131 w134] -> w128
              frame 2 {
                n421 = Enqueue Element(queue=w132, element=CameraControlTypeDef."Idle" ("Enum")) -> (queue out=w131:refnum<queue>)  [unwired: 2 in, 2 out]
              }
              frame 1, Default {
                n422 = Enqueue Element(queue=w135, element=CameraControlTypeDef."Preview" ("Enum")) -> (queue out=w134:refnum<queue>)  [unwired: 2 in, 2 out]
              }
            }
            n423 = Enqueue Element(queue=w128, element=CameraControlTypeDef."Update" ("Enum")) -> ()  [unwired: 2 in, 3 out]
          }
          event "Trigger Mode": Value Change {
            n424 = event-data() -> ("NewVal"=w137:sgl)  [unwired: 1 in, 5 out]
            n425 = case shown="6" w137 {
              tunnel: w139 -> [w142 w145]
              tunnel: [w141 w144] -> w138
              frame 6 {
                n426 = Enqueue Element(queue=w142, element=CameraControlTypeDef."Idle" ("Enum")) -> (queue out=w141:refnum<queue>)  [unwired: 2 in, 2 out]
              }
              frame 1, Default {
                n427 = Enqueue Element(queue=w145, element=CameraControlTypeDef."Preview" ("Enum")) -> (queue out=w144:refnum<queue>)  [unwired: 2 in, 2 out]
              }
            }
            n428 = Enqueue Element(queue=w138, element=CameraControlTypeDef."Trigger Mode" ("Enum")) -> ()  [unwired: 2 in, 3 out]
          }
          event "Internal Line Interval": Value Change {
            n429 = event-data() -> ("OldVal"=w148:dbl)  [unwired: 1 in, 5 out]
            n430 = Enqueue Element(queue=w149, element=CameraControlTypeDef."IntervalLineInt", timeout in ms (-1)=w148) -> ()  [unwired: 1 in, 3 out]
          }
        }
      }
      n431 = call <userlib>:"tm_stopcapture.vi"("error in (no error)"=w22, "Handle in"=w23) -> ("error out"=w69:errorcluster, "Handle out"=w70:u32)  [unwired: 8 in]
      n432 = call <userlib>:"tm_unpreparecapture.vi"("error in (no error)"=w69, "Handle in"=w70) -> ("error out"=w68:errorcluster, "Handle out"=w71:u32)  [unwired: 8 in]
      n433 = call <userlib>:"tm_closecamera.vi"("error in (no error)"=w68, "Handle in"=w71) -> ("error out"=w96:errorcluster)  [unwired: 9 in]
      n434 = call <userlib>:"tm_deinitialize.vi"("error in (no error)"=w96) -> ("error out"=w18:errorcluster)  [unwired: 10 in]
      n435 = Release Queue(queue=w17, error in (no error)=w18) -> (error out=w16:errorcluster)  [unwired: 1 in, 2 out]
      n436 = Release Queue(queue=w14, error in (no error)=w16) -> (error out=w15:errorcluster)  [unwired: 1 in, 2 out]
    }
  }
  "error out" <- w3
